vi "VASP Helper.vi"() -> ()   [LabVIEW 2010]
uses:
  <vilib>/Utility/miscctls.llb/LV3DPointTypeDef.ctl
  <vilib>/addons/database/_DB Variant To Data/Database Variant To Data.xnode
  <vilib>/Analysis/6fits.llb/Curve Fitting Criteria.ctl
  <vilib>/Analysis/_algsub.llb/Real Vector Norm.vi
  <vilib>/Utility/file.llb/Read From Spreadsheet File (string).vi
  <vilib>/addons/database/Connection.llb/DB Tools Open Connec (Path).vi
  <vilib>/gmath/NumericalOptimization/Nonlinear Curve Fit LM formula string.vi
  <vilib>/Utility/file.llb/Write To Spreadsheet File (string).vi
  <vilib>/Analysis/NI_AALPro.lvlib
  <vilib>/addons/database/NI_Database_API.lvlib
  <vilib>/picture/3D Picture Control/NI_3D Picture Control.lvlib
  <vilib>/gmath/NI_Gmath.lvlib
panel:
  in  "Bulk Stds":T1(array[cluster])=[{"Bulk Name"="Relax2", "Structure ID"="i8VcOVQciOra", "Final Energy (eV)"=-19.916802, "Atom Counts"=[{"Atomic Species"="Cd", "Total Count"=4}, {"Atomic Species"="Te", "Total Count"=4}]}, {"Bulk Name"="Gamma8_64atom", "Structure ID"="KHRErLzu78i1", "Final Energy (eV)"=-159.32149, "Atom Counts"=[{"Atomic Species"="Cd", "Total Count"=32}, {"Atomic Species"="Te", "Total Count"=32}]}, {"Bulk Name"="Gamma8_216atom", "Structure ID"="LhCMwqUcPen4", "Final Energy (eV)"=-537.73861, "Atom Counts"=[{"Atomic Species"="Cd", "Total Count"=108}, {"Atomic Species"="Te", "Total Count"=108}]}, {"Bulk Name"="Gamma8_111Bulk", "Structure ID"="Ku1Zi1Vogv1V", "Final Energy (eV)"=-29.865487, "Atom Counts"=[{"Atomic Species"="Cd", "Total Count"=6}, {"Atomic Species"="Te", "Total Count"=6}]}, {"Bulk Name"="A3B3_Supercell_C+0.147672", "Structure ID"="F1CSD7Lr82d2", "Final Energy (eV)"=-358.27975, "Atom Counts"=[{"Atomic Species"="Cd", "Total Count"=72}, {"Atomic Species"="Te", "Total Count"=72}]}, {"Bulk Name"="A4B1_Supercell_C+0.130973", "Structure ID"="gulg5TYIiUnY", "Final Energy (eV)"=-298.52824, "Atom Counts"=[{"Atomic Species"="Cd", "Total Count"=60}, {"Atomic Species"="Te", "Total Count"=60}]}]
  out "IDs":T2
  out "Temp Interfacial Area":dbl
  out "Temp # of atoms":i32
  out "Temp Values":string[](array[string])
  out "Temp Headers":string[](array[string])
  out "Using DB":bool
  out "Selected DOS":T3
  out "DOS Array":T4(array[cluster])
  out "Selected Structure":T5
  out "PickPoint":T6
  out "DOS Plot Names":string[](array[string])
  out "Saved DOS Plots":cluster{dbl[], dbl[]}[](array[cluster])
  in  "Plot Formation Energy":bool
  in  "Plot Band Edge Diagram":bool=TRUE
  in  "Plot Bivariate":bool=TRUE
  in  "Save Summary":bool
  in  "Plot Structures":bool
  in  "Primary Path":path
  in  "Clean Cache":bool
  in  "Loaded DFT Paths":path[](array[path])
  out "OSZICAR Raw Array":T7(array[cluster])
  out "All DFT Data Summary":T8
  in  "Plot Relaxation":bool
  in  "Plot DOS":bool
  in  "Plot Variability":bool
  in  "Load from DB":bool
  in  "Load from Directory":bool
  in  "Details":i32[](listbox)
  in  "Selection List":i32[](listbox)
  in  "Tab Control":T9(tab)
  out "Overview DOS PLot":cluster{dbl[], dbl[]}[](graph)
  out "Overview - Relaxation":cluster{"Formation Energy (eV)":dbl[]}[](graph)
  out "Overview - Parameter Analysis Graph":cluster{"Voltage":dbl[], dbl[]}[](graph)=[{"Voltage"=[], []}, {"Voltage"=[1.0], [nan]}]
  out "Relaxation":cluster{"Formation Energy (eV)":dbl[]}[](graph)
  in  "Relaxation Y-Axis":string(combo)="Energy"
  in  "Send to DOS":bool
  in  "Load in VESTA":bool
  in  "Auto Setup Camera":bool
  out "Atomic Structure":refnum<vi>(3d-picture)
  in  "Animate Relaxation":bool
  in  "Atom Size":dbl=0.75
  in  "# Frames":i32(slide)=5 scale=0.0..100.0
  in  "Atom List":i32[](listbox)
  in  "Scale":dbl(slide)=0.07482993197278912 scale=0.0..0.5
  in  "CONTCAR?":bool
  in  "Look at Atoms":bool
  in  "Plot Name":string
  in  "Erase":bool
  in  "DOS Sum and Plot":bool
  in  "DOS Options":i32[](listbox)
  in  "Always Show Bulk":bool
  out "DOS PLot":cluster{dbl[], dbl[]}[](graph)
  in  "S Orbitals":bool
  in  "P Orbital":bool
  in  "D Orbitals":bool
  out "Band Edge Diagram":cluster{"Array":dbl[], dbl[]}[](graph)
  in  "Low Density Cutoff":dbl
  in  "Style":enum16{"Linear Step", "Linear Pts", "Log Pts"}(ring)
  in  "Step or #pts":dbl
  in  "Grouping Columns":u16[](array[ring])=[2] items=["Full_Directory", "Parent_Folder", "Folder", "# Atoms", "Cell Volume (A^3)", "|A| (Å)", "|B| (Å)", "|C| (Å)", "alpha (deg)", "beta (deg)", "gamma (deg)", "Final_Energy_(eV)", "Final Energy/atom (eV/atom)", "Total Formation Energy (eV)", "E0 at Sigma=0 (eV)", "dE (eV)", "Interfacial Energy (J/m²)", "Calc Time (hrs)", "Grain 1 Orientation", "Grain 2 Orientation", "Twist Angle (Degree)", "Tilt Angle (Degree)", "Translation (x,y,z)", "Overlap Length (A)", "Grain 1 Start (A)", "Defect Name", "Location"]
  in  "Parameter Analysis Y-Axis":u16(ring)=23 caption="| Current Density | (A/cm2)" items=["Full_Directory", "Parent_Folder", "Folder", "# Atoms", "Cell Volume (A^3)", "|A| (Å)", "|B| (Å)", "|C| (Å)", "alpha (deg)", "beta (deg)", "gamma (deg)", "Final_Energy_(eV)", "Final Energy/atom (eV/atom)", "Total Formation Energy (eV)", "E0 at Sigma=0 (eV)", "dE (eV)", "Interfacial Energy (J/m²)", "Calc Time (hrs)", "Grain 1 Orientation", "Grain 2 Orientation", "Twist Angle (Degree)", "Tilt Angle (Degree)", "Translation (x,y,z)", "Overlap Length (A)", "Grain 1 Start (A)", "Defect Name", "Location"]
  out "Parameter Analysis Graph":cluster{"Voltage":dbl[], dbl[]}[](graph)=[{"Voltage"=[], []}, {"Voltage"=[1.0], [nan]}]
  in  "model description":T10
  out "best fit parameters":dbl[](array[numeric])
  in  "initial parameters":dbl[](array[numeric])
  out "R²":dbl
  out "X_min":dbl
  in  "Bivariate X-Axis":string(combo)="Energy"
  in  "Bivariate Y-Axis":string(combo)="Energy"
  out "Bivariate Plot":cluster{dbl[], dbl[]}[](graph)
  out "Ymin":dbl
  out "Polynomial Coefficients":dbl[](array[numeric])
  in  "Standard Bulk Calculations":i32[](listbox)
  in  "Add to point defect DB":bool
  out "Te Rich Limit":cluster{"appended array":dbl[], dbl[]}[](graph)
  out "Reference Energy (eV)":dbl format="%#_6f"
  out "Cd Rich Limit":cluster{"appended array":dbl[], dbl[]}[](graph)
  in  "Add to README files":bool
  in  "Loaded Files":i32[](listbox)
  in  "Size Factor":i32=1
  out "GB Bivariate Plot":cluster{dbl[], dbl[]}(graph)
  in  "Interface Free Reference Energy":i32[](listbox)
  in  "GB Size Factor":dbl=1.0
  out "GB Reference Energy (eV)":dbl
  in  "Add to GB DB":bool
  in  "Color Array Type":T11(ring)=enum."Contrasting Colors"
  in  "Load Energies":bool=TRUE
  in  "Load DOS":bool=TRUE
  in  "Only total DOS":bool=TRUE
  out "Structures":T12(array[cluster])
  out "All Available DFT Paths":path[](array[path])
  in  "Vesta .exe Location":path=path "C:/Program Files (x86)/VESTA/VESTA.exe"
  out "Selectd Defect Data":T13(array[cluster])
  out "Base Object":refnum<vi>
  in  "Vasp DB UDL":path=path "D:/Ab-initio/VASP Calcs/VASP DB.udl"
  in  "Options":cluster{"Border?":bool, "Bonds?":bool}={"Border?"=TRUE, "Bonds?"=FALSE}
  # "After"
  # "Before"
  # "You need non self-cons"
  # "Most Specific"
  # "Least Specific"
  # "Interface at b*c"
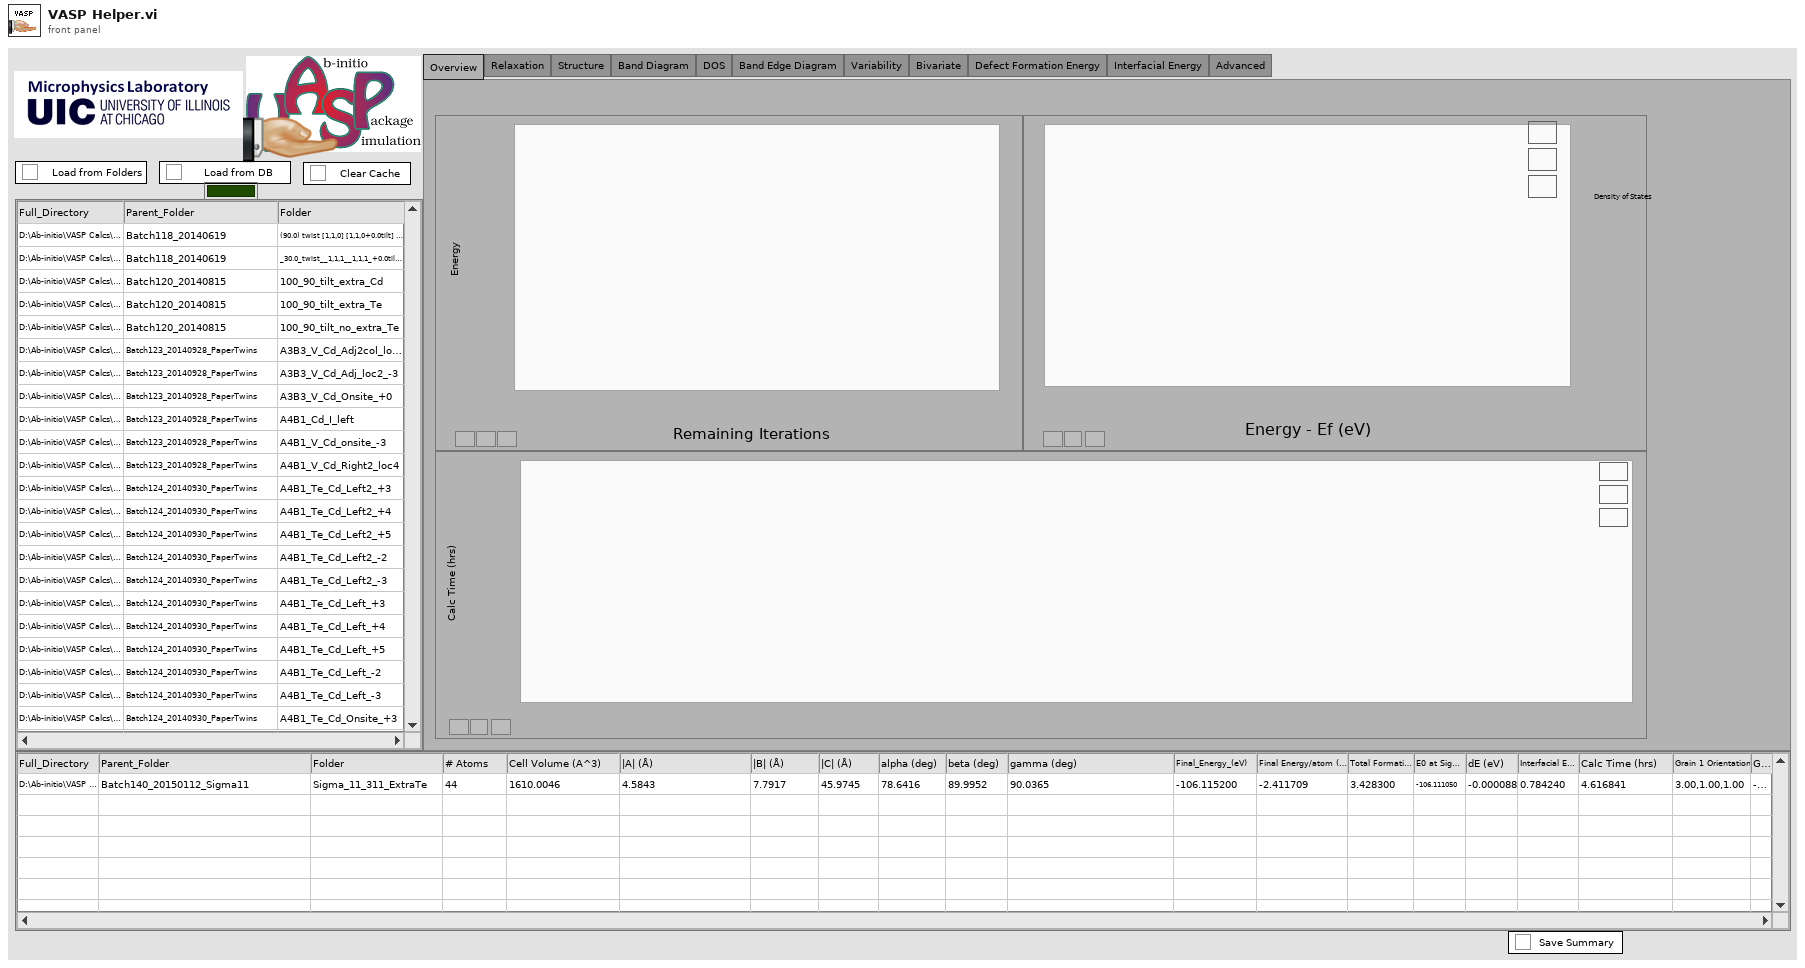
[diagram p1: front panel]
types:
  T1 = cluster{"Bulk Name":string, "Structure ID":string, "Final Energy (eV)":dbl, "Atom Counts":cluster{"Atomic Species":string, "Total Count":i32}[]}[]
  T2 = cluster{"CONTCAR ID":string, "OSZICAR ID":string, "DOSCAR ID":string}
  T3 = cluster{"DOS Summary":cluster{"Fermi Level (eV)":dbl, "# Filled States":dbl, "Density of Valence Band":dbl, "Density of Condution Band":dbl}, "Total DOS":cluster{"Energy (eV)":dbl[], "Total DOS":dbl[], "Integrated DOS":dbl[]}, "Atomic-decomposed DOS":cluster{"Fermi Level (eV)":dbl, "# of Filled States":dbl, "DOS":dbl[][]}[]}
  T4 = cluster{"DOS Summary":cluster{"Fermi Level (eV)":dbl, "# Filled States":dbl, "Density of Valence Band":dbl, "Density of Condution Band":dbl}, "Total DOS":cluster{"Energy (eV)":dbl[], "Total DOS":dbl[], "Integrated DOS":dbl[]}, "Atomic-decomposed DOS":cluster{"Fermi Level (eV)":dbl, "# of Filled States":dbl, "DOS":dbl[][]}[]}[]
  T5 = cluster{"Structure Name":string, "Lattice vector a":dbl[], "Lattice vector b":dbl[], "Lattice vector c":dbl[], "Atoms Array":cluster{"Atom Name":string, "Positions (Direct)":dbl[][], "Positions (Cartesian)":dbl[][]}[], "# of atoms":i32}
  T6 = typedef "LV3DPointTypeDef.ctl" = cluster{"X":sgl, "Y":sgl, "Z":sgl}
  T7 = cluster{"OSZICAR data":cluster{"Total Free Energy (eV)":dbl, "E0 at Sigma=0 (eV)":dbl, "dE (eV)":dbl, "Electronic Relaxation":dbl[][]}[], "Ionic Relaxation Energies Array (eV)":dbl[], "Bulk Formation Energies Array (eV)":dbl[]}[]
  T8 = cluster{"Headers":string[], "Relaxation Data":string[][]}
  T9 = enum32{"Overview", "Relaxation", "Structure", "Band Diagram", "DOS", "Band Edge Diagram", "Variability", "Bivariate", "Defect Formation Energy", "Interfacial Energy", "Advanced"}
  T10 = cluster{"model":string, "Parameters":string[], "x":string}
  T11 = enum16{"Visible Spectrum", "Greyscale", "Contrasting Colors"}
  T12 = cluster{"Structure Name":string, "Lattice vector a":dbl[], "Lattice vector b":dbl[], "Lattice vector c":dbl[], "Atoms Array":cluster{"Atom Name":string, "Positions (Direct)":dbl[][], "Positions (Cartesian)":dbl[][]}[], "# of atoms":i32}[]
  T13 = cluster{"Final Total Defect Energy (eV)":dbl, "Reference Pure Structure Energy":dbl, "N (Cd,Ideal - Cd,Defect)":i32, "N (Te,ideal - Te,defect)":i32, "# Extra Electrons":i32}[]
  T14 = cluster{"DOS Summary":cluster{"Fermi Level (eV)":dbl, "# States":dbl, "Density of Valence Band":dbl, "Density of Condution Band":dbl}, "Total DOS":cluster{"Energy (eV)":dbl[], "Total DOS":dbl[], "Integrated DOS":dbl[]}, "Atomic-decomposed DOS":cluster{"Fermi Level (eV)":dbl, "# of Filled States":dbl, "DOS":dbl[][]}[]}[]
  T15 = enum32{"Overview", "Relaxation", "Structure", "Band Diagram", "DOS", "Band Edge Diagram", "Variability", "Bivariate", "Defect Formation Energy", "Advanced"}
  T16 = cluster{"OSZICAR data":cluster{"Total Free Energy (eV)":dbl, "E0 at Sigma=0 (eV)":dbl, "dE (eV)":dbl, "Electronic Relaxation":dbl[][]}[], "Ionic Relaxation Energies Array (eV)":dbl[], "Bulk Formation Energies Array (eV)":dbl[]}
  T17 = cluster{"Final Energy (eV)":dbl, "Final Energy/atom (eV/atom)":dbl, "Total Formation Energy (eV)":dbl}
  T18 = cluster{"Fermi Level (eV)":dbl, "# of Filled States":dbl, "DOS":dbl[][]}[]
  T19 = cluster{"Energy (eV)":dbl[], "Total DOS":dbl[], "Integrated DOS":dbl[]}
  T20 = cluster{"Fermi Level (eV)":dbl, "# States":dbl, "Density of Valence Band":dbl, "Density of Condution Band":dbl}
  T21 = cluster{"DOS Summary":cluster{"Fermi Level (eV)":dbl, "# States":dbl, "Density of Valence Band":dbl, "Density of Condution Band":dbl}, "Total DOS":cluster{"Energy (eV)":dbl[], "Total DOS":dbl[], "Integrated DOS":dbl[]}, "Atomic-decomposed DOS":cluster{"Fermi Level (eV)":dbl, "# of Filled States":dbl, "DOS":dbl[][]}[]}
  T22 = typedef "NI_Database_API.lvlib/Conn ObjectReference.ctl" = refnum<k1>
  T23 = cluster{"[0]":string, "[1]":string, "[2]":string}
  T24 = cluster{"Bulk Formation Energies Array (eV)":dbl[]}
  T25 = cluster{"Atom Name":string, "Positions (Direct)":dbl[][], "Positions (Cartesian)":dbl[][]}[]
  T26 = cluster{"Fermi Level (eV)":dbl, "# of Filled States":dbl, "DOS":dbl[][]}
  T27 = typedef "NI_AALPro.lvlib/Curve Fitting Criteria.ctl" = u16
  T28 = cluster{"Lattice vector b[0]":dbl, "Lattice vector b[1]":dbl, "Lattice vector b[2]":dbl}
  T29 = typedef "LVPoint32TypeDef.ctl" = cluster{"Horizontal":i32, "Vertical":i32}
  T30 = cluster{"Shift":bool, "Ctrl":bool, "Alt":bool, "Cmd":bool, "Opt":bool}
  T31 = typedef "LVPositionTypeDef.ctl" = cluster{"Left":i32, "Top":i32}
  T32 = cluster{"Bulk Name":string, "Structure ID":string, "Final Energy (eV)":dbl, "Atom Counts":cluster{"Atomic Species":string, "Total Count":i32}[]}
  T33 = cluster{"Atomic Species":string, "Total Count":i32}[]
  T34 = cluster{"String":string, string, dbl, "Atom Counts":cluster{"Atomic Species":string, "Total Count":i32}[]}
  T35 = cluster{"Atomic Species":string, "Total Count":i32}
  T36 = cluster{"String":string, "Site Density":dbl, dbl, i32, i32}
  T37 = cluster{cluster{"String":string, "Site Density":dbl, dbl, i32, i32}, cluster{string, string, "Net Charge":i32, dbl}[]}
  T38 = cluster{"String":string, "Structure ID":string, "String":string, "String":string, i32, "Structure ID":string, "name":string, "Reference Pure Structure Energy":dbl, "N (Cd,Ideal - Cd,Defect)":i32, "N (Te,ideal - Te,defect)":i32, string}
  T39 = cluster{"DFT ID":string, "Structure ID":string, "Defect_Name":string, "Location":string, "Net Charge":i32, "Defect Free Structure ID":string, "Defect Free Structure Name":string, "Reference Pure Structure Energy":dbl, "N Mising Cd":i32, "N Missing Te":i32, "Comments":string}[]
  T40 = cluster{"MD5 message-digest":string, "Structure ID":string, "String":string, "Structure ID":string, "name":string, "GB Reference Energy (eV)":dbl, "t":dbl, dbl, dbl, "String":string, string}
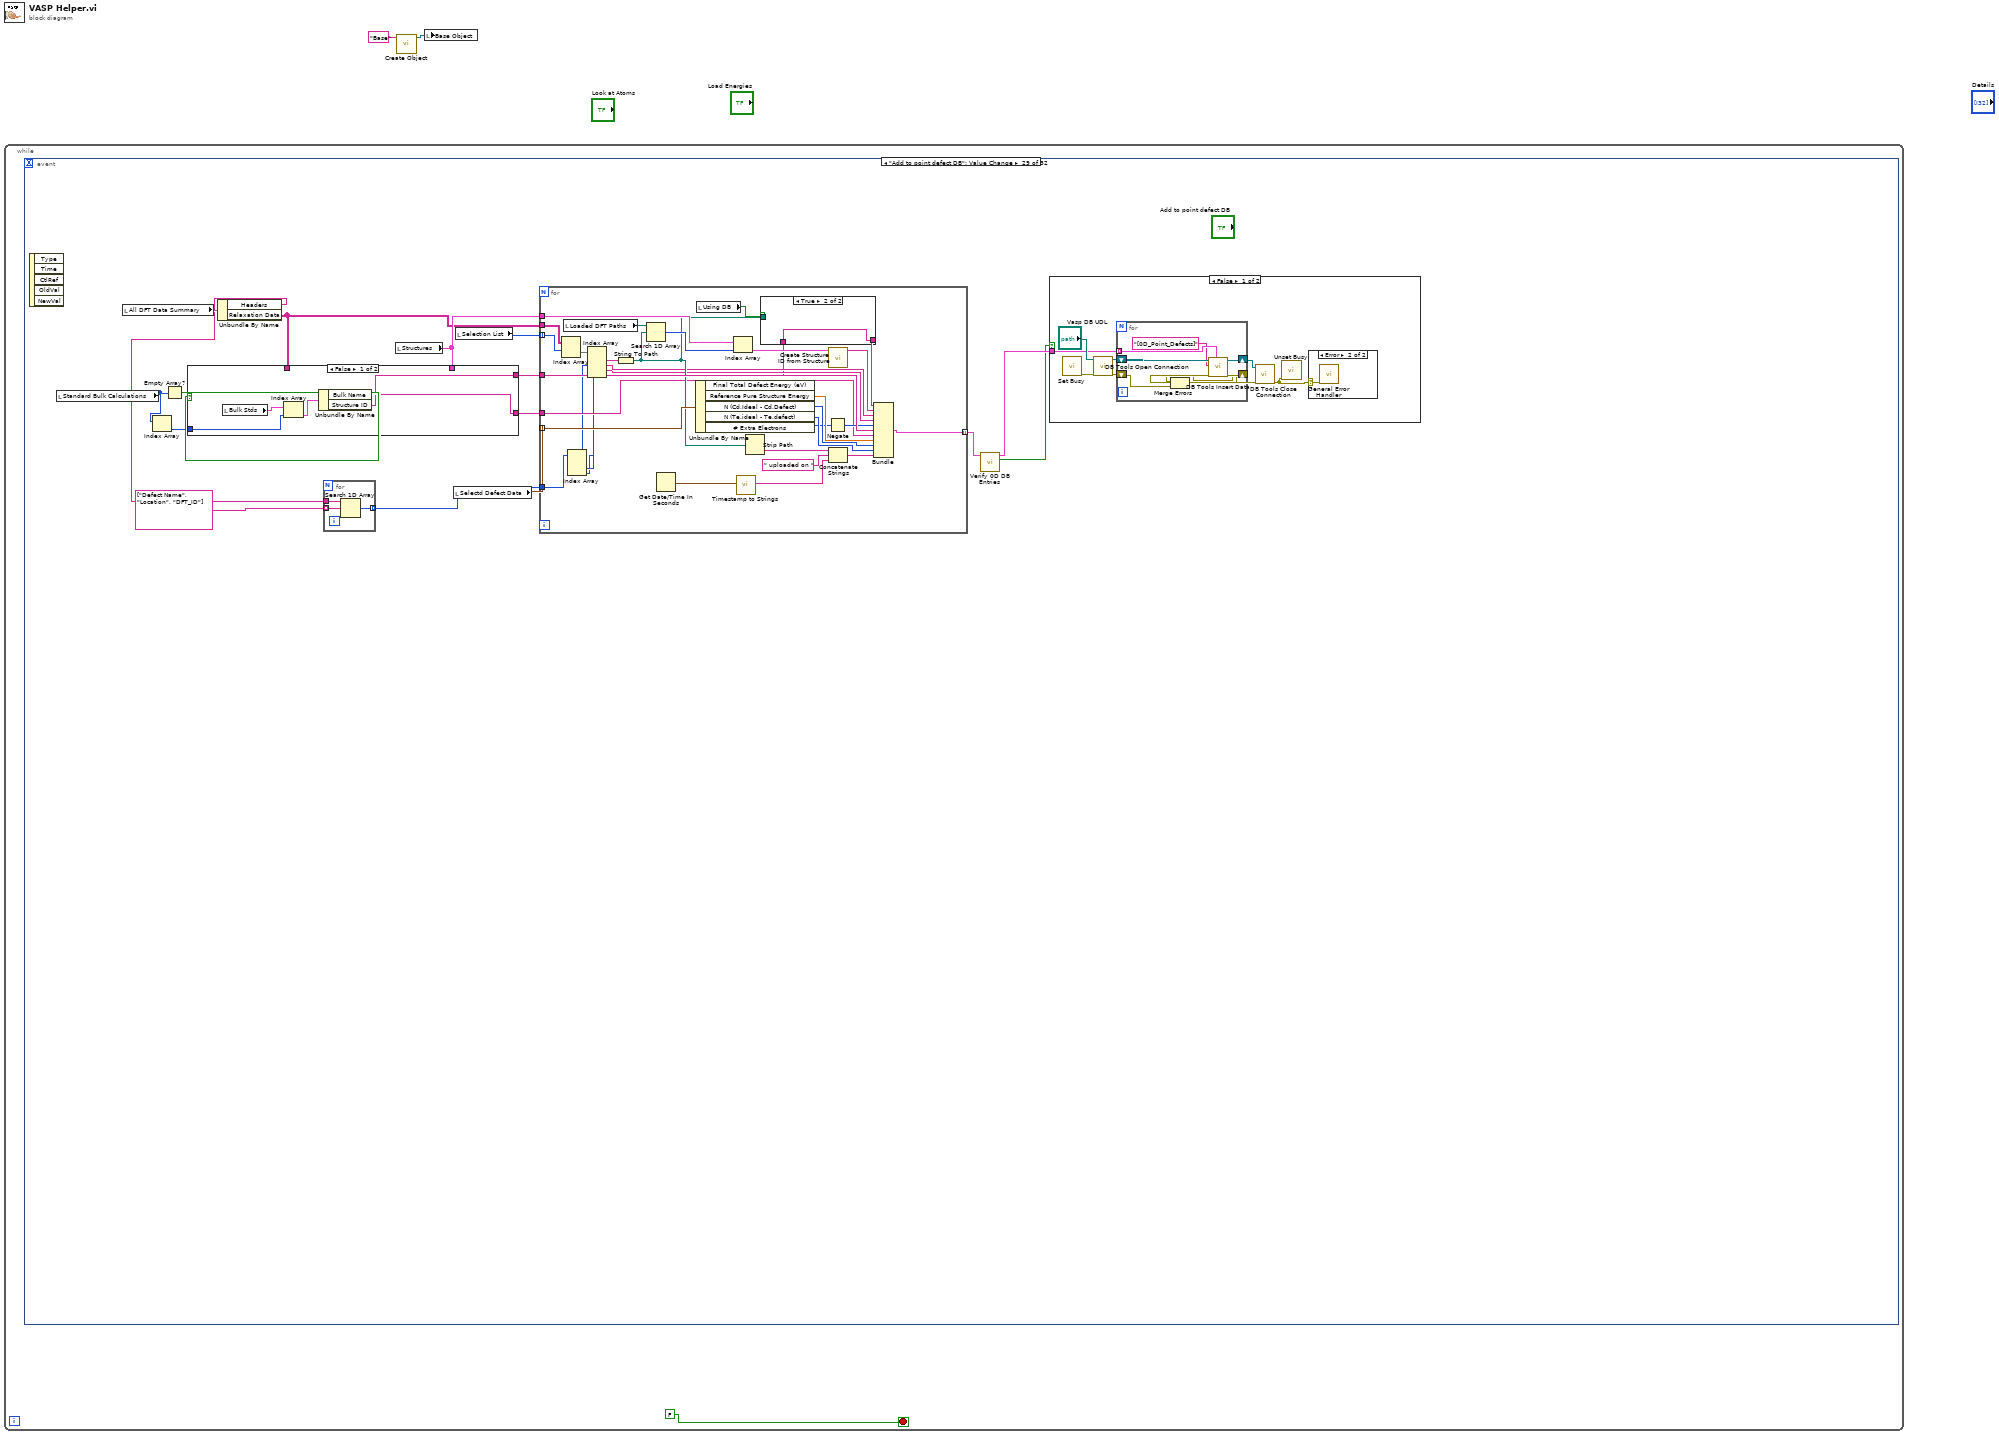
[diagram p0: block diagram]
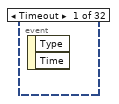
[diagram p2: hidden frame]
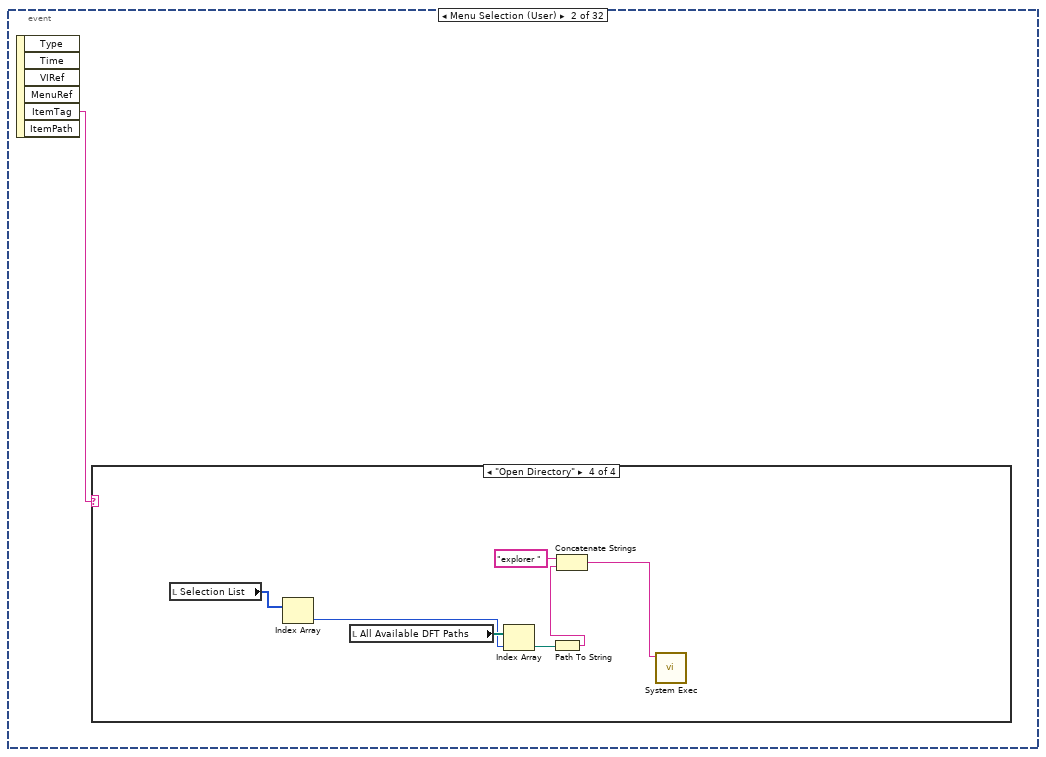
[diagram p3: hidden frame]
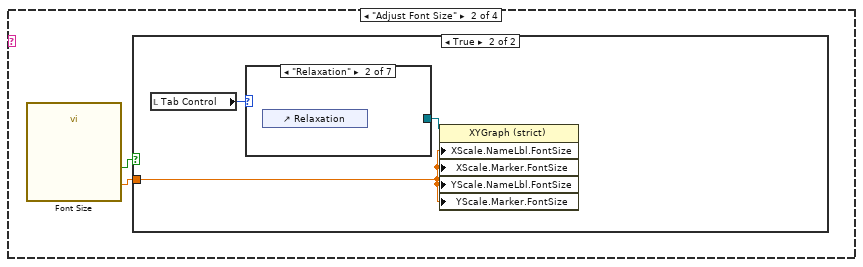
[diagram p5: hidden frame]
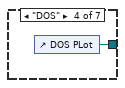
[diagram p9: hidden frame]
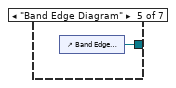
[diagram p10: hidden frame]
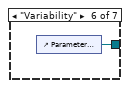
[diagram p11: hidden frame]
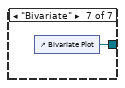
[diagram p12: hidden frame]
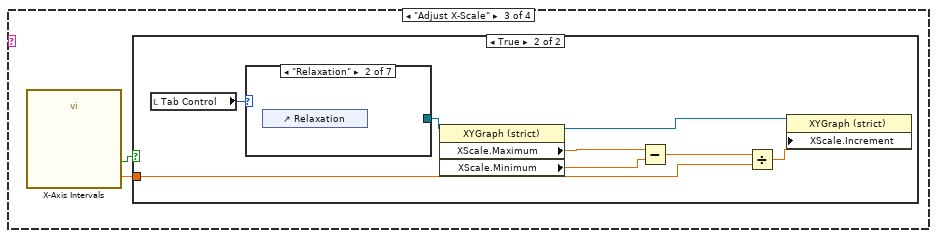
[diagram p13: hidden frame]
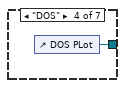
[diagram p17: hidden frame]
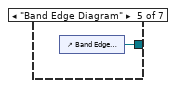
[diagram p18: hidden frame]
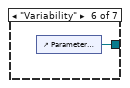
[diagram p19: hidden frame]
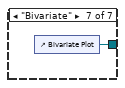
[diagram p20: hidden frame]
diagram:
  n1 = while {
    stop <- FALSE stop-if-true
    n2 = event shown="[28] \"Add to point defect DB\": Value Change" {
      selector: _ -> [_ _ _ _ _ _ _ _ _ _ _ _ _ _ _ _ _ _ _ _ _ _ _ _ _ _ _ _ _ _ _ _]
      dyn-events: _ -> [_ _ _ _ _ _ _ _ _ _ _ _ _ _ _ _ _ _ _ _ _ _ _ _ _ _ _ _ _ _ _ _]
      timeout: _ -> [_ _ _ _ _ _ _ _ _ _ _ _ _ _ _ _ _ _ _ _ _ _ _ _ _ _ _ _ _ _ _ _]
      event Timeout {
        n3 = event-data() -> ()  [unwired: 1 in, 2 out]
      }
      event Menu Selection (User) {
        n4 = event-data() -> ("ItemTag"=w4:string)  [unwired: 1 in, 5 out]
        n5 = case shown="\"Open Directory\"" w4 {
          frame Default {
          }
          frame "Adjust Font Size" {
            n6 = call "Font Size"() -> ("Font Size"=w5:dbl, "Apply"=w6:bool)  [unwired: 17 in, 1 out]
            n7 = case shown="True" w6 {
              tunnel: w5 -> [_ w9]
              frame False {
              }
              frame True {
                n8 = local read "Tab Control"() -> (w8:T9)
                n9 = case shown="\"Relaxation\"" w8 {
                  tunnel: [_ _ _ w10 w11 w12 w13] -> w7
                  frame "Overview", Default {
                  }
                  frame "Relaxation" {
                    n10 = control-ref of="Relaxation"() -> ()  [unwired: 1 out]
                  }
                  frame "Structure" {
                  }
                  frame "DOS" {
                    n11 = control-ref of="DOS PLot"() -> (w10:refnum<vi>)
                  }
                  frame "Band Edge Diagram" {
                    n12 = control-ref of="Band Edge Diagram"() -> (w11:refnum<vi>)
                  }
                  frame "Variability" {
                    n13 = control-ref of="Parameter Analysis Graph"() -> (w12:refnum<vi>)
                  }
                  frame "Bivariate" {
                    n14 = control-ref of="Bivariate Plot"() -> (w13:refnum<vi>)
                  }
                }
                n15 = property on="Property Node" class="XYGraph (strict)"(reference=w7, "XScale.NameLbl.FontSize"=w9, "XScale.Marker.FontSize"=w9, "YScale.NameLbl.FontSize"=w9, "YScale.Marker.FontSize"=w9) -> ()  [unwired: 1 in, 2 out]
              }
            }
          }
          frame "Adjust X-Scale" {
            n16 = call "X-Axis Intervals"() -> ("# Intervals"=w14:dbl, "Apply"=w15:bool)  [unwired: 17 in, 1 out]
            n17 = case shown="True" w15 {
              tunnel: w14 -> [_ w19]
              frame False {
              }
              frame True {
                n18 = local read "Tab Control"() -> (w23:T9)
                n19 = case shown="\"Relaxation\"" w23 {
                  tunnel: [_ _ _ w24 w25 w26 w27] -> w17
                  frame "Overview", Default {
                  }
                  frame "Relaxation" {
                    n20 = control-ref of="Relaxation"() -> ()  [unwired: 1 out]
                  }
                  frame "Structure" {
                  }
                  frame "DOS" {
                    n21 = control-ref of="DOS PLot"() -> (w24:refnum<vi>)
                  }
                  frame "Band Edge Diagram" {
                    n22 = control-ref of="Band Edge Diagram"() -> (w25:refnum<vi>)
                  }
                  frame "Variability" {
                    n23 = control-ref of="Parameter Analysis Graph"() -> (w26:refnum<vi>)
                  }
                  frame "Bivariate" {
                    n24 = control-ref of="Bivariate Plot"() -> (w27:refnum<vi>)
                  }
                }
                n25 = property on="Property Node" class="XYGraph (strict)"(reference=w17) -> (reference out=w16:refnum<vi>, "XScale.Maximum"=w22:dbl, "XScale.Minimum"=w21:dbl)  [unwired: 1 in, 1 out]
                n26 = Subtract(x=w22, y=w21) -> (x-y=w20:dbl)
                n27 = Divide(x=w20, y=w19) -> (x/y=w18:dbl)
                n28 = property on="Property Node" class="XYGraph (strict)"(reference=w16, "XScale.Increment"=w18) -> ()  [unwired: 1 in, 2 out]
              }
            }
          }
          frame "Open Directory" {
            n29 = local read "Selection List"() -> (w33:i32[])
            n30 = Index Array(array=w33) -> (element=w32:i32)  [unwired: 1 in]
            n31 = local read "All Available DFT Paths"() -> (w34:path[])
            n32 = Index Array(array=w34, index=w32) -> (element=w28:path)
            n33 = Path To String(path=w28) -> (string=w31:string)
            n34 = Concatenate Strings("explorer " ("string"), w31) -> (w29:string)
            n35 = call <vilib>:"System Exec.vi"("command line"=w29) -> ()  [unwired: 7 in, 4 out]
          }
        }
      }
      event "Primary Path", "Load from Directory": Value Change {
        w35 = string[] ["Full_Directory", "Parent_Folder", "Folder"]
        n36 = event-data() -> ()  [unwired: 1 in, 5 out]
        n37 = call "File Dialog2"("start path"=path "D:/Ab-initio/VASP Calcs" ("Folder Path"), "prompt"="Please choose the primary path where all VASP calculation folders are stored.\nThis will be done recursively") -> ("selected path"=w40:path)  [unwired: 10 in, 3 out]
        n38 = flat-sequence {
          frame #0 {
            n39 = local write "Loaded DFT Paths"(path[] [] ("Loaded DFT Paths")) -> ()
            n40 = local write "OSZICAR Raw Array"(T7 [] ("OSZICAR Raw Array")) -> ()
            n41 = local write "DOS Array"(T14 [] ("DOS Array")) -> ()
            n42 = local write "Structures"(T12 [] ("Structures")) -> ()
            n43 = Request Deallocation(TRUE ("flag")) -> ()
          }
        }
        n44 = local write "Primary Path"(w40) -> ()
        n45 = call <vilib>:"Recursive File List.vi"("Folder Path"=w40) -> ("All Folders"=w45:path[])  [unwired: 6 in, 4 out]
        n46 = for {
          tunnel: w45 -> [w55] mode=indexing
          shift-right: [w54] -> w41
          shift-left: path[] [] -> [w53]
          shift-right: [w52] -> w36
          shift-left: string[][] [] -> [w51]
          n47 = Build Path(base path=w55, name or relative path="POSCAR") -> (appended path=w57:path)
          n48 = call <vilib>:"Check if File or Folder Exists.vi"("path"=w57) -> ("file or folder exists?"=w56:bool)  [unwired: 8 in, 2 out]
          n49 = case shown="False" w56 {
            tunnel: w55 -> [_ w67]
            tunnel: [w60 w70] -> w54
            tunnel: w53 -> [w60 w69]
            tunnel: [w59 w62] -> w52
            tunnel: w51 -> [w59 w61]
            frame False {
            }
            frame True {
              n50 = Build Array (concatenate)(w69, w67) -> (w70:path[])
              n51 = Strip Path(path=w67) -> (stripped path=w66:path, name=w65:string)
              n52 = Path To String(path=w67) -> (string=w68:string)
              n53 = Strip Path(path=w66) -> (name=w64:string)  [unwired: 1 out]
              n54 = Build Array(w68, w64, w65) -> (w63:string[])
              n55 = Build Array (concatenate)(w61, w63) -> (w62:string[][])
            }
          }
        }
        "All Available DFT Paths" <- w41
        n56 = local write "Using DB"(FALSE ("Using DB")) -> ()
        n57 = property on="Selection List" class="MCListbox (strict)"("ColHdrString"=w35, "ItemNames"=w36) -> ()  [unwired: 2 in, 2 out]
        n58 = Bundle(w35, w36) -> (w42:cluster{string[], string[][]})  [unwired: 1 in]
        n59 = local write "All DFT Data Summary"(w42) -> ()
        n60 = property on="Loaded Files" class="MCListbox (strict)"("ItemNames"=w36) -> ()  [unwired: 2 in, 2 out]
        n61 = property on="Interface Free Reference Energy" class="MCListbox (strict)"("ColHdrString"=w35, "ItemNames"=w36) -> ()  [unwired: 2 in, 2 out]
      }
      event "Load from DB": Value Change {
        n62 = event-data() -> ()  [unwired: 1 in, 5 out]
        n63 = flat-sequence {
          frame #0 {
            n64 = local write "Loaded DFT Paths"(path[] [] ("Loaded DFT Paths")) -> ()
            n65 = local write "OSZICAR Raw Array"(T7 [] ("OSZICAR Raw Array")) -> ()
            n66 = local write "DOS Array"(T14 [] ("DOS Array")) -> ()
            n67 = local write "Structures"(T12 [] ("Structures")) -> ()
            n68 = Request Deallocation(TRUE ("flag")) -> ()
          }
        }
        n69 = call "Import from VASP DB.vi"() -> ("error out"=w74:errorcluster, "All DFT Data Summary"=w78:T8)  [unwired: 10 in]
        n70 = local write "All DFT Data Summary"(w78) -> ()
        n71 = Unbundle(w78) -> ("Headers"=w71:string[], "Relaxation Data"=w72:string[][])
        n72 = property on="Selection List" class="MCListbox (strict)"("ColHdrString"=w71, "ItemNames"=w72) -> ()  [unwired: 2 in, 2 out]
        n73 = property on="Loaded Files" class="MCListbox (strict)"("ItemNames"=w72) -> ()  [unwired: 2 in, 2 out]
        n74 = property on="Details" class="MCListbox (strict)"("ColHdrString"=w71) -> ()  [unwired: 2 in, 2 out]
        n75 = Index Array(array=w72, index (col)=0 ("disabled index (col)")) -> (element=w76:string[])  [unwired: 1 in]
        n76 = for {
          tunnel: w76 -> [w85] mode=indexing
          tunnel: [w84] -> w75 mode=indexing
          tunnel: w74 -> [_]
          n77 = String To Path(string=w85) -> (path=w84:path)
        }
        n78 = property on="Interface Free Reference Energy" class="MCListbox (strict)"("ColHdrString"=w71, "ItemNames"=w72) -> ()  [unwired: 2 in, 2 out]
        n79 = local write "All Available DFT Paths"(w75) -> ()
        "Using DB" <- TRUE ("Using DB")
      }
      event "Selection List": Value Change {
        n80 = event-data() -> ()  [unwired: 1 in, 5 out]
        n81 = for {
          tunnel: [w98] -> w86 mode=indexing
          tunnel: "Selection List" -> [w95] mode=indexing
          tunnel: [w92] -> w87
          n82 = local read "All Available DFT Paths"() -> (w93:path[])
          n83 = Index Array(array=w93, index=w95) -> (element=w96:path)
          n84 = Search 1D Array(1D array="Loaded DFT Paths", element=w96) -> (index of element=w97:i32)  [unwired: 1 in]
          n85 = case shown="-1" w97 {
            tunnel: [w100 w106] -> w98
            tunnel: w96 -> [_ w107]
            tunnel: w95 -> [w101 w108]
            tunnel: [w99 w105] -> w92
            frame Default {
              n86 = local read "All DFT Data Summary"() -> (w103:T8)
              n87 = Unbundle By Name(w103) -> ("Headers"=w99:string[], "Relaxation Data"=w102:string[][])
              n88 = Index Array(array=w102, index (row)=w101) -> (element=w100:string[])  [unwired: 1 in]
            }
            frame -1 {
              n89 = local read "Using DB"() -> (w104:bool)
              n90 = case shown="True" w104 {
                tunnel: w108 -> [w112 w222]
                tunnel: w107 -> [w111 w225]
                tunnel: [w110 w223] -> w106
                tunnel: [w109 w224] -> w105
                frame False {
                  n91 = stacked-sequence {
                    tunnel: w112 -> [_ _ _ _ _ _ _ w213]
                    tunnel: w111 -> [w115 w119 w141 w166 w176 w179 w199 _]
                    tunnel: [_ _ _ _ _ _ _ w209] -> w110
                    tunnel: [_ _ _ _ _ _ _ w210] -> w109
                    tunnel: [_ _ _ _ w168 _ _ _] -> _
                    frame #0 {
                      w113 = string[] [] ("Temp Headers")
                      # "Add new path to list"
                      n92 = local read "Loaded DFT Paths"() -> (w116:path[])
                      n93 = local write "Temp Headers"(w113) -> ()
                      n94 = local write "Temp Values"(w113) -> ()
                      n95 = Build Array (concatenate)(w116, w115) -> (w114:path[])
                      n96 = local write "Loaded DFT Paths"(w114) -> ()
                    }
                    frame #1 {
                      n97 = Strip Path(path=w119) -> (stripped path=w127:path, name=w124:string)
                      n98 = Path To String(path=w119) -> (string=w126:string)
                      n99 = Strip Path(path=w127) -> (name=w125:string)  [unwired: 1 out]
                      n100 = Build Array(w126, w125, w124) -> (w121:string[])
                      n101 = local read "Temp Headers"() -> (w123:string[])
                      n102 = local read "Temp Values"() -> (w122:string[])
                      n103 = Build Array (concatenate)(w123, string[] ["Full_Directory", "Parent_Folder", "Folder"]) -> (→"Temp Headers":string[])
                      n104 = Build Array (concatenate)(w122, w121) -> (→"Temp Values":string[])
                    }
                    frame #2 {
                      n105 = Build Path(base path=w141, name or relative path="CONTCAR") -> (appended path=w144:path)
                      n106 = call "Parse POSCAR.vi"("POSCAR File"=w144) -> ("Summary Values"=w136:string[], "Summary Headers"=w137:string[], "Structure"=w131:T5)  [unwired: 7 in, 1 out]
                      n107 = Unbundle By Name(w131) -> ("Lattice vector a"=w134:dbl[], "Lattice vector b"=w133:dbl[], "# of atoms"=→"Temp # of atoms":i32)
                      n108 = local read "Temp Headers"() -> (w138:string[])
                      n109 = local read "Temp Values"() -> (w140:string[])
                      n110 = local read "Structures"() -> (w142:T12)
                      n111 = call <vilib>:"Cross Product.vi"("B Vector"=w133, "A Vector"=w134) -> ("Cross Product"=w132:dbl[])  [unwired: 8 in, 1 out]
                      n112 = call-poly <vilib>:"Vector Norm.vi"("Input Vector"=w132) -> ("norm"=→"Temp Interfacial Area":dbl)  [unwired: 9 in, 1 out]
                      n113 = Build Array (concatenate)(w142, w131) -> (→"Structures":T12)
                      n114 = Build Array (concatenate)(w138, w137) -> (w135:string[])
                      n115 = Build Array (concatenate)(w140, w136) -> (w139:string[])
                      n116 = local write "Temp Headers"(w135) -> ()
                      n117 = local write "Temp Values"(w139) -> ()
                    }
                    frame #3 {
                      w149 = 2.0  # # of interfaces
                      w154 = 16.0217656  # Unit Conversion
                      n118 = local read "Temp # of atoms"() -> (w156:i32)
                      n119 = local read "OSZICAR Raw Array"() -> (w163:T7)
                      n120 = local read "Temp Headers"() -> (w160:string[])
                      n121 = Build Path(base path=w166, name or relative path="OSZICAR") -> (appended path=w165:path)
                      n122 = call "Parse OSZICAR (Energies).vi"("# of Atoms"=w156, "OSZICAR File"=w165) -> ("Summary Values"=w157:string[], "Summary Headers"=w158:string[], "OSZICAR Raw"=w164:T16, "Extracted Parameters"=w153:T17)  [unwired: 6 in]
                      n123 = Unbundle By Name(w153) -> ("Total Formation Energy (eV)"=w152:dbl)
                      n124 = Build Array (concatenate)(w160, w158, "Interfacial Energy (J/m²)") -> (w159:string[])
                      n125 = Build Array (concatenate)(w163, w164) -> (→"OSZICAR Raw Array":T7)
                      n126 = local read "Temp Interfacial Area"() -> (w151:dbl)
                      n127 = local write "Temp Headers"(w159) -> ()
                      n128 = Divide(x=w152, y=w151) -> (x/y=w155:dbl)
                      n129 = Multiply(x=w154, y=w155) -> (x*y=w150:dbl)
                      n130 = Divide(x=w150, y=w149) -> (x/y=w148:dbl)
                      n131 = local read "Temp Values"() -> (w162:string[])
                      n132 = Number To Fractional String(number=w148) -> (F-format string=w147:string)  [unwired: 3 in]
                      n133 = Build Array (concatenate)(w162, w157, w147) -> (w161:string[])
                      n134 = local write "Temp Values"(w161) -> ()
                    }
                    frame #4 {
                      n135 = local read "Temp Headers"() -> (w174:string[])
                      n136 = Build Path(base path=w176, name or relative path="OUTCAR") -> (appended path=w177:path)
                      n137 = call "Parse OUTCAR.vi"("OUTCAR File"=w177) -> ("error out"=w168:errorcluster, "Calc Time (Hrs)"=w171:dbl)  [unwired: 8 in, 1 out]
                      n138 = local read "Temp Values"() -> (w172:string[])
                      n139 = Build Array (concatenate)(w174, "Calc Time (hrs)") -> (w175:string[])
                      n140 = Number To Fractional String(number=w171) -> (F-format string=w169:string)  [unwired: 3 in]
                      n141 = local write "Temp Headers"(w175) -> ()
                      n142 = Build Array (concatenate)(w172, w169) -> (w173:string[])
                      n143 = local write "Temp Values"(w173) -> ()
                    }
                    frame #5 {
                      n144 = case shown="True" "Load DOS" {
                        tunnel: w179 -> [_ w189]
                        tunnel: [_ w188] -> _
                        tunnel: [_ w184] -> w182
                        frame False {
                        }
                        frame True {
                          n145 = Build Path(base path=w189, name or relative path="DOSCAR") -> (appended path=w191:path)
                          n146 = call "Parse DOSCAR.vi"("Only total DOS"="Only total DOS", "Path"=w191) -> ("error out"=w188:errorcluster, "Atomic-decomposed DOS"=w185:T18, "Total DOS"=w186:T19, "DOS Summary"=w187:T20)  [unwired: 6 in]
                          n147 = Bundle("DOS Summary"=w187, "Total DOS"=w186, "Atomic-decomposed DOS"=w185) -> (w184:T21)  [unwired: 1 in]
                        }
                      }
                      n148 = local read "DOS Array"() -> (w180:T4)
                      n149 = Build Array (concatenate)(w180, w182) -> (→"DOS Array":T14)
                    }
                    frame #6 {
                      n150 = Build Path(base path=w199, name or relative path="README.txt") -> (appended path=w201:path)
                      n151 = call <vilib>:"Check if File or Folder Exists.vi"("path"=w201) -> ("file or folder exists?"=w200:bool)  [unwired: 8 in, 2 out]
                      n152 = case shown="True" w200 {
                        tunnel: w201 -> [_ w207]
                        tunnel: [_ w204] -> w194
                        tunnel: [_ w203] -> w193
                        frame False {
                        }
                        frame True {
                          n153 = call-poly <vilib>:"Read From Spreadsheet File.vi"("file path (dialog if empty)"=w207) -> ("all rows"=w206:string[][])  [unwired: 6 in, 4 out]
                          n154 = Index Array(array=w206, index (col) #1=0 ("disabled index (col)")) -> (element #1=w204:string[], element #2=w203:string[])  [unwired: 3 in]
                        }
                      }
                      n155 = local read "Temp Headers"() -> (w197:string[])
                      n156 = local read "Temp Values"() -> (w195:string[])
                      n157 = Build Array (concatenate)(w197, w194) -> (w198:string[])
                      n158 = Build Array (concatenate)(w195, w193) -> (w196:string[])
                      n159 = local write "Temp Headers"(w198) -> ()
                      n160 = local write "Temp Values"(w196) -> ()
                    }
                    frame #7 {
                      n161 = local read "All DFT Data Summary"() -> (w211:T8)
                      n162 = Unbundle By Name(w211) -> ("Headers"=w221:string[], "Relaxation Data"=w214:string[][])
                      n163 = local read "Temp Headers"() -> (w219:string[])
                      n164 = local read "Temp Values"() -> (w218:string[])
                      n165 = Index Array(array=w214, index (row)=w213) -> (element=w220:string[])  [unwired: 1 in]
                      n166 = call "Updated Dynamic Headers.vi"("Old Data"=w220, "New Data"=w218, "This Data's Headers"=w219, "Old Headers"=w221) -> ("Formatted New Data"=w209:string[], "Merged Headers"=w210:string[])  [unwired: 6 in]
                      n167 = Build Array (concatenate)(w209, w214) -> (w217:string[][])
                      n168 = Delete From Array(array=w217, index (row)=0) -> (array with subset deleted=w215:string[][])  [unwired: 2 in, 1 out]
                      n169 = Replace Array Subset(array=w215, new element=w209, index (row)=w213) -> (w212:string[][])  [unwired: 1 in]
                      n170 = Bundle By Name(cluster=w211, "Headers"=w210, "Relaxation Data"=w212) -> (→"All DFT Data Summary":T8)
                    }
                  }
                }
                frame True {
                  n171 = local read "Vasp DB UDL"() -> (w226:path)
                  n172 = call-poly <vilib>:"DB Tools Open Connection.vi"("connection information"=w226) -> ("connection reference"=w227:T22)  [unwired: 7 in, 1 out]
                  n173 = stacked-sequence {
                    tunnel: w227 -> [_ w233 _ w267 w308 w312 _]
                    tunnel: w225 -> [w228 w232 _ w261 _ _ _]
                    tunnel: [_ _ w252 _ _ _ _] -> w224
                    tunnel: [_ _ w251 _ _ _ _] -> w223
                    tunnel: w222 -> [_ w231 w250 _ _ _ _]
                    frame #0 {
                      n174 = local read "Loaded DFT Paths"() -> (w230:path[])
                      n175 = Build Array (concatenate)(w230, w228) -> (w229:path[])
                      n176 = local write "Loaded DFT Paths"(w229) -> ()
                    }
                    frame #1 {
                      # "No need to update"
                      n177 = disable-structure shown="Disabled" {
                        disable-tunnel: w233 -> [w249 _]
                        disable-tunnel: w232 -> [w248 _]
                        disable-tunnel: [w243 _] -> _
                        disable-tunnel: [w242 _] -> _
                        disable-tunnel: w231 -> [w237 _]
                        frame Disabled {
                          n178 = local read "All DFT Data Summary"() -> (w240:T8)
                          n179 = Unbundle By Name(w240) -> ("Headers"=w241:string[], "Relaxation Data"=w235:string[][])
                          n180 = call "Query Headers and Data from VASP DB.vi"("Full Path"=w248, "connection reference"=w249) -> ("Data"=w242:string[], "Headers"=w243:string[])  [unwired: 6 in, 2 out]
                          n181 = Index Array(array=w235, index (row)=w237) -> (element=w236:string[])  [unwired: 1 in]
                          n182 = call "Updated Dynamic Headers.vi"("Old Data"=w236, "New Data"=w242, "This Data's Headers"=w243, "Old Headers"=w241) -> ("Formatted New Data"=w244:string[], "Merged Headers"=w239:string[])  [unwired: 6 in]
                          n183 = Build Array (concatenate)(w235, w244) -> (w247:string[][])
                          n184 = Delete From Array(array=w247, index (row)=0) -> (array with subset deleted=w245:string[][])  [unwired: 2 in, 1 out]
                          n185 = Replace Array Subset(array=w245, new element=w244) -> (w234:string[][])  [unwired: 2 in]
                          n186 = Bundle By Name(cluster=w240, "Headers"=w239, "Relaxation Data"=w234) -> (w238:T8)
                          n187 = local write "All DFT Data Summary"(w238) -> ()
                        }
                        frame Enabled {
                        }
                      }
                    }
                    frame #2 {
                      n188 = local read "All DFT Data Summary"() -> (w254:T8)
                      n189 = Unbundle By Name(w254) -> ("Headers"=w252:string[], "Relaxation Data"=w253:string[][])
                      n190 = Index Array(array=w253, index (row)=w250) -> (element=w251:string[])  [unwired: 1 in]
                    }
                    frame #3 {
                      n191 = Path To String(path=w261) -> (string=w260:string)
                      n192 = Concatenate Strings("WHERE Full_Directory ='", w260, "'" ("string")) -> (w262:string)
                      n193 = call <vilib>:"DB Tools Select Data.vi"("condition"=w262, "columns"=string[] ["CONTCAR_Structure_ID", "OSZICAR_ID", "DOSCAR_ID"], "table"="DFT_Summary", "connection reference"=w267) -> ("data"=w259:variant[][])  [unwired: 2 in, 2 out]
                      n194 = Index Array(array=w259, index (row)=0) -> (element=w257:variant[])  [unwired: 1 in]
                      n195 = for {
                        tunnel: w257 -> [w270] mode=indexing
                        tunnel: [w268] -> w256 mode=indexing
                        n196 = xnode "Database Variant To Data"("database variant"=w270, "type"="") -> ("data"=w268:string)  [unwired: 1 in, 1 out]
                      }
                      n197 = Array To Cluster(array=w256) -> (cluster=→"IDs":T23)
                    }
                    frame #4 {
                      n198 = local read "IDs"() -> (w306:T2)
                      n199 = Unbundle By Name(w306) -> ("CONTCAR ID"=w305:string)
                      n200 = call "Import Structure from DB.vi"("Structure ID"=w305, "connection reference"=w308) -> ("Loaded Structure"=w304:T5)  [unwired: 7 in, 2 out]
                      n201 = local read "Structures"() -> (w309:T12)
                      n202 = Unbundle By Name(w304) -> ("# of atoms"=w303:i32)
                      n203 = Build Array (concatenate)(w309, w304) -> (w307:T12)
                      n204 = local write "Temp # of atoms"(w303) -> ()
                      n205 = local write "Structures"(w307) -> ()
                    }
                    frame #5 {
                      n206 = local read "IDs"() -> (w315:T2)
                      n207 = local read "Temp # of atoms"() -> (w314:i32)
                      n208 = Unbundle By Name(w315) -> ("OSZICAR ID"=w313:string)
                      n209 = local read "OSZICAR Raw Array"() -> (w316:T7)
                      n210 = call "Import Energies (OSZICAR) from DB.vi"("# of Atoms"=w314, "OSZICAR ID"=w313, "connection reference"=w312) -> ("OSZICAR Raw"=w311:T16)  [unwired: 5 in, 3 out]
                      n211 = Build Array (concatenate)(w316, w311) -> (w310:T7)
                      n212 = local write "OSZICAR Raw Array"(w310) -> ()
                    }
                    frame #6 {
                      n213 = disable-structure shown="Disabled" {
                        frame Disabled {
                          n214 = local read "DOS Array"() -> (w318:T4)
                          n215 = local read "IDs"() -> (w317:T2)
                          n216 = local read "Only total DOS"() -> ()  [unwired: 1 out]
                          n217 = Unbundle By Name(w317) -> ()  [unwired: 1 out]
                          n218 = Build Array (concatenate)(w318) -> ()  [unwired: 1 in, 1 out]
                        }
                        frame Enabled {
                        }
                      }
                    }
                  }
                }
              }
            }
          }
        }
        n219 = call <vilib>:"Set Busy.vi"() -> ("error out"=w88:errorcluster)  [unwired: 10 in, 1 out]
        n220 = property on="Bivariate Y-Axis" class="CmbBox"("Strings[]"=w87) -> ()  [unwired: 2 in, 2 out]
        n221 = property on="Grouping Col List" class="Ring (strict)"("Strings []"=w87) -> ()  [unwired: 2 in, 2 out]
        n222 = property on="Bivariate X-Axis" class="CmbBox"("Strings[]"=w87) -> ()  [unwired: 2 in, 2 out]
        n223 = property on="Parameter Analysis Y-Axis" class="Ring (strict)"("Strings []"=w87) -> ()  [unwired: 2 in, 2 out]
        n224 = property on="Details" class="MCListbox (strict)"(error in=w88, "ColHdrString"=w87, "ItemNames"=w86) -> (error out=w89:errorcluster)  [unwired: 1 in, 1 out]
        n225 = case shown="\"Interfacial Energy\"" "Tab Control" {
          tunnel: w89 -> [_ _ _ _ _ _ _ _ _]
          frame "Overview", Default {
            n226 = property on="Plot Relaxation" class="Bool (strict)"("Val(Sgnl)"=TRUE ("Value (Signaling)")) -> ()  [unwired: 2 in, 2 out]
            n227 = property on="Plot DOS" class="Bool (strict)"("Val(Sgnl)"=TRUE ("Value (Signaling)")) -> ()  [unwired: 2 in, 2 out]
            n228 = property on="Plot Variability" class="Bool (strict)"("Val(Sgnl)"=TRUE ("Value (Signaling)")) -> ()  [unwired: 2 in, 2 out]
          }
          frame "Relaxation" {
            n229 = property on="Plot Relaxation" class="Bool (strict)"("Val(Sgnl)"=TRUE ("Value (Signaling)")) -> ()  [unwired: 2 in, 2 out]
          }
          frame "Structure" {
            n230 = property on="Plot Structures" class="Bool (strict)"("Val(Sgnl)"=TRUE ("Value (Signaling)")) -> ()  [unwired: 2 in, 2 out]
          }
          frame "DOS" {
            n231 = property on="Plot DOS" class="Bool (strict)"("Val(Sgnl)"=TRUE ("Value (Signaling)")) -> ()  [unwired: 2 in, 2 out]
          }
          frame "Variability" {
            n232 = property on="Plot Variability" class="Bool (strict)"("Val(Sgnl)"=TRUE ("Value (Signaling)")) -> ()  [unwired: 2 in, 2 out]
          }
          frame "Bivariate" {
            n233 = property on="Plot Bivariate" class="Bool (strict)"("Val(Sgnl)"=TRUE ("Value (Signaling)")) -> ()  [unwired: 2 in, 2 out]
          }
          frame "Band Edge Diagram" {
            n234 = property on="Plot Band Edge Diagram" class="Bool (strict)"("Val(Sgnl)"=TRUE ("Value (Signaling)")) -> ()  [unwired: 2 in, 2 out]
          }
          frame "Defect Formation Energy" {
            n235 = property on="Plot Formation Energy" class="Bool (strict)"("Val(Sgnl)"=TRUE ("Value (Signaling)")) -> ()  [unwired: 2 in, 2 out]
          }
          frame "Interfacial Energy" {
            n236 = local read "GB Size Factor"() -> (w329:dbl)
            n237 = property on="GB Size Factor" class="DigNum (strict)"("Val(Sgnl)"=w329) -> ()  [unwired: 2 in, 2 out]
          }
        }
        n238 = call <vilib>:"Unset Busy.vi"("error in (no error)"=w89) -> ()  [unwired: 10 in, 1 out]
      }
      event "Plot Relaxation": Value Change {
        n239 = event-data() -> ()  [unwired: 1 in, 5 out]
        n240 = local read "All DFT Data Summary"() -> (w331:T8)
        n241 = Unbundle By Name(w331) -> ("Relaxation Data"=w330:string[][])
        n242 = local read "Selection List"() -> (w337:i32[])
        n243 = for {
          tunnel: w337 -> [w365] mode=indexing
          tunnel: [w361] -> w334 mode=indexing
          tunnel: [w366] -> w332 mode=indexing
          tunnel: w330 -> [w357]
          n244 = Index Array(array=w357, index (row)=w365) -> (element=w364:string[])  [unwired: 1 in]
          n245 = local read "Loaded DFT Paths"() -> (w356:path[])
          n246 = Index Array(array=w364, index #2=2 ("index"), index #3=3 ("index")) -> (element #1=w363:string, element #2=w361:string, element #3=w359:string)  [unwired: 1 in]
          n247 = local read "OSZICAR Raw Array"() -> (w353:T7)
          n248 = String To Path(string=w363) -> (path=w355:path)
          n249 = Decimal String To Number(string=w359) -> (number=w358:i32)  [unwired: 2 in, 1 out]
          n250 = Search 1D Array(1D array=w356, element=w355) -> (index of element=w354:i32)  [unwired: 1 in]
          n251 = Index Array(array=w353, index=w354) -> (element=w352:T16)
          n252 = case shown="\"Formation Energy/Atom\"" "Relaxation Y-Axis" {
            tunnel: w352 -> [w370 w372 w376 w380]
            tunnel: [w369 w373 w377 w379] -> w367
            tunnel: w358 -> [_ w374 w378 _]
            frame "Energy", Default {
              n253 = Unbundle By Name(w370) -> ("Ionic Relaxation Energies Array (eV)"=w369:dbl[])
            }
            frame "Energy/Atom" {
              n254 = Unbundle By Name(w372) -> ("Ionic Relaxation Energies Array (eV)"=w371:dbl[])
              n255 = Divide(x=w371, y=w374) -> (x/y=w373:dbl[])
            }
            frame "Formation Energy/Atom" {
              n256 = Unbundle By Name(w376) -> ("Bulk Formation Energies Array (eV)"=w375:dbl[])
              n257 = Divide(x=w375, y=w378) -> (x/y=w377:dbl[])
            }
            frame "Formation Energy" {
              n258 = Unbundle By Name(w380) -> ("Bulk Formation Energies Array (eV)"=w379:dbl[])
            }
          }
          n259 = Bundle("Bulk Formation Energies Array (eV)"=w367) -> (w366:T24)  [unwired: 1 in]
        }
        "Relaxation" <- w332
        "Overview - Relaxation" <- w332
        n260 = Array Size(array=w334) -> (size(s)=w333:i32)
        n261 = local read "Color Array Type"() -> (w336:T11)
        n262 = call "Num of Colors to Color Array.vi"("# of Colors"=w333, "Color Array Type"=w336) -> ("Colors Array"=w335:u32[])  [unwired: 3 in]
        n263 = for {
          N -> [w343]
          tunnel: w334 -> [w342] mode=indexing
          tunnel: w335 -> [w341] mode=indexing
          i -> [w344]
          n264 = control-ref of="Relaxation"() -> (w339:refnum<vi>)
          n265 = control-ref of="Overview - Relaxation"() -> (w340:refnum<vi>)
          n266 = Build Array(w339, w340) -> (w338:refnum<vi>[])
          n267 = for {
            tunnel: w344 -> [w351]
            tunnel: w343 -> [w350]
            tunnel: w342 -> [w349]
            tunnel: w341 -> [w347]
            tunnel: w338 -> [w345] mode=indexing
            n268 = property on="Property Node" class="WFGraph (strict)"(reference=w345, "Active Plot"=w351, "LegNumRows"=w350, "Plot.Plot Name"=w349, "Plot.Point Style"=u8 2, "Plot.Fill/Pt. Color"=w347, "Plot.Plot Interpolation"=u8 0) -> ()  [unwired: 1 in, 2 out]
          }
        }
      }
      event "Relaxation Y-Axis": Value Change {
        n269 = event-data() -> ("NewVal"=w381:string)  [unwired: 1 in, 4 out]
        n270 = property on="Relaxation" class="WFGraph (strict)"("YScale.NameLbl.Text"=w381) -> ()  [unwired: 2 in, 2 out]
        n271 = property on="Overview - Relaxation" class="WFGraph (strict)"("YScale.NameLbl.Text"=w381) -> ()  [unwired: 2 in, 2 out]
        n272 = property on="Plot Relaxation" class="Bool (strict)"("Val(Sgnl)"=TRUE ("Value (Signaling)")) -> ()  [unwired: 2 in, 2 out]
      }
      event "Tab Control": Value Change {
        n273 = event-data() -> ("NewVal"=w383:T9)  [unwired: 1 in, 4 out]
        n274 = case shown="\"Overview\", Default" w383 {
          frame "Overview", Default {
            (unwired) 0 ("Value (Signaling)")
            n275 = property on="Plot Relaxation" class="Bool (strict)"("Val(Sgnl)"=TRUE ("Value (Signaling)")) -> ()  [unwired: 2 in, 2 out]
            n276 = property on="Plot Variability" class="Bool (strict)"("Val(Sgnl)"=TRUE ("Value (Signaling)")) -> ()  [unwired: 2 in, 2 out]
            n277 = property on="Plot DOS" class="Bool (strict)"("Val(Sgnl)"=TRUE ("Value (Signaling)")) -> ()  [unwired: 2 in, 2 out]
          }
          frame "Relaxation" {
            n278 = property on="Plot Relaxation" class="Bool (strict)"("Val(Sgnl)"=TRUE ("Value (Signaling)")) -> ()  [unwired: 2 in, 2 out]
          }
          frame "Structure" {
            n279 = property on="Plot Structures" class="Bool (strict)"("Val(Sgnl)"=TRUE ("Value (Signaling)")) -> ()  [unwired: 2 in, 2 out]
          }
          frame "DOS" {
            n280 = property on="Plot DOS" class="Bool (strict)"("Val(Sgnl)"=TRUE ("Value (Signaling)")) -> ()  [unwired: 2 in, 2 out]
          }
          frame "Variability" {
            n281 = property on="Plot Variability" class="Bool (strict)"("Val(Sgnl)"=TRUE ("Value (Signaling)")) -> ()  [unwired: 2 in, 2 out]
          }
          frame "Bivariate" {
            n282 = property on="Plot Bivariate" class="Bool (strict)"("Val(Sgnl)"=TRUE ("Value (Signaling)")) -> ()  [unwired: 2 in, 2 out]
          }
          frame "Defect Formation Energy" {
            n283 = property on="Plot Formation Energy" class="Bool (strict)"("Val(Sgnl)"=TRUE ("Value (Signaling)")) -> ()  [unwired: 2 in, 2 out]
          }
        }
      }
      event "Plot DOS", "Always Show Bulk": Value Change {
        n284 = event-data() -> ()  [unwired: 1 in, 5 out]
        n285 = local read "All DFT Data Summary"() -> (w414:T8)
        n286 = local read "Selection List"() -> (w411:i32[])
        n287 = Unbundle By Name(w414) -> ("Relaxation Data"=w413:string[][])
        n288 = Index Array(array=w411) -> (element=w410:i32)  [unwired: 1 in]
        n289 = Index Array(array=w413, index (row)=w410) -> (element=w409:string[])  [unwired: 1 in]
        n290 = local read "Loaded DFT Paths"() -> (w406:path[])
        n291 = Index Array(array=w409, index #2=2 ("index")) -> (element #1=w408:string, element #2=w399:string)  [unwired: 1 in]
        n292 = String To Path(string=w408) -> (path=w405:path)
        n293 = Build Array (concatenate)(w399, "Total DOS" ("element"), string[] ["", "", "", "", "", "", ""] ("appended array")) -> (w398:string[])
        n294 = local read "DOS Array"() -> (w404:T4)
        n295 = local read "Structures"() -> (w403:T12)
        n296 = Search 1D Array(1D array=w406, element=w405) -> (index of element=w402:i32)  [unwired: 1 in]
        n297 = Index Array(array=w403, index=w402) -> (element=w401:T5)
        n298 = Index Array(array=w404, index=w402) -> (element=→"Selected DOS":T3)
        n299 = Unbundle By Name(w401) -> ("Atoms Array"=w400:T25)
        n300 = Build Array(w398) -> (w396:string[][])
        n301 = for {
          tunnel: w400 -> [w423] mode=indexing
          shift-right: [w419] -> w412
          shift-left: w396 -> [w418]
          tunnel: w399 -> [w417]
          n302 = Unbundle By Name(w423) -> ("Atom Name"=w420:string, "Positions (Direct)"=w422:dbl[][], "Positions (Cartesian)"=w421:dbl[][])
          n303 = for {
            tunnel: w422 -> [w432] mode=indexing
            tunnel: w421 -> [w431] mode=indexing
            tunnel: w420 -> [w430]
            shift-right: [w426] -> w419
            shift-left: w418 -> [w425]
            tunnel: w417 -> [w424]
            n304 = Number To Fractional String(number=w432) -> (F-format string=w429:string[])  [unwired: 3 in]
            n305 = Number To Fractional String(number=w431) -> (F-format string=w428:string[])  [unwired: 3 in]
            n306 = Build Array (concatenate)(w424, w430, w429, w428) -> (w427:string[])
            n307 = Build Array (concatenate)(w425, w427) -> (w426:string[][])
          }
        }
        n308 = property on="DOS Options" class="MCListbox (strict)"("ItemNames"=w412) -> (error out=w394:errorcluster)  [unwired: 2 in, 1 out]
        n309 = disable-structure shown="Disabled" {
          disable-tunnel: w394 -> [w415 _]
          frame Disabled {
            n310 = property on="DOS Options" class="MCListbox (strict)"(error in=w415, "Val(Sgnl)"=i32[] [0] ("Value (Signaling)")) -> ()  [unwired: 1 in, 2 out]
          }
          frame Enabled {
          }
        }
      }
      event "DOS Options": Value Change {
        n311 = event-data() -> ()  [unwired: 1 in, 5 out]
        n312 = local read "Selected DOS"() -> (w436:T3)
        n313 = Unbundle By Name(w436) -> ("DOS Summary.Fermi Level (eV)"=w439:dbl, "DOS Summary.# Filled States"=w434:dbl)
        n314 = Unbundle By Name(w436) -> ("Total DOS.Energy (eV)"=w438:dbl[])
        n315 = Subtract(x=w438, y=w439) -> (x-y=w437:dbl[])
        n316 = Array Size(array=w438) -> (size(s)=w440:i32)
        n317 = Initialize Array(0.0 ("Numeric"), w440) -> (w448:dbl[])
        n318 = for {
          tunnel: "DOS Options" -> [w462] mode=indexing
          shift-right: [w459] -> w435
          shift-left: w448 -> [w460]
          tunnel: w436 -> [w461]
          n319 = case shown="0" w462 {
            selector: w462 -> [_ w476]
            tunnel: w461 -> [w464 w478]
            tunnel: w460 -> [_ w468]
            tunnel: [w463 w465] -> w459
            frame 0 {
              n320 = Unbundle By Name(w464) -> ("Total DOS.Total DOS"=w463:dbl[])
            }
            frame 1, Default {
              n321 = Unbundle By Name(w478) -> ("Atomic-decomposed DOS"=w477:T18)
              n322 = Decrement(x=w476) -> (x-1=w475:i32)
              n323 = Index Array(array=w477, index=w475) -> (element=w474:T26)
              n324 = Build Array(FALSE ("element"), "S Orbitals", "P Orbital", "P Orbital", "P Orbital", "D Orbitals", "D Orbitals", "D Orbitals", "D Orbitals", "D Orbitals") -> (w469:bool[])
              n325 = Unbundle By Name(w474) -> ("DOS"=w473:dbl[][])
              n326 = Transpose 2D Array(2D array=w473) -> (transposed array=w472:dbl[][])
              n327 = for {
                shift-right: [w480] -> w465
                shift-left: w468 -> [w479]
                tunnel: w472 -> [w482] mode=indexing
                tunnel: w469 -> [w481] mode=indexing
                n328 = case shown="False" w481 {
                  tunnel: w482 -> [_ w486]
                  tunnel: [w483 w485] -> w480
                  tunnel: w479 -> [w483 w484]
                  frame False {
                  }
                  frame True {
                    n329 = Add(x=w486, y=w484) -> (x+y=w485:dbl[])
                  }
                }
              }
            }
          }
        }
        n330 = local read "DOS Plot Names"() -> (w445:string[])
        n331 = Build Array (concatenate)("Current", w445) -> (w443:string[])
        n332 = Array Size(array=w443) -> (size(s)=w458:i32)
        n333 = call "Num of Colors to Color Array.vi"("# of Colors"=w458, "Color Array Type"="Color Array Type") -> ("Colors Array"=w455:u32[])  [unwired: 3 in]
        n334 = Divide(x=w435, y=w434) -> (x/y=w433:dbl[])
        n335 = Bundle(w437, w433) -> (w447:cluster{dbl[], dbl[]})  [unwired: 1 in]
        n336 = case shown="True" "Always Show Bulk" {
          tunnel: [w487 w500] -> w446
          tunnel: [w489 w498] -> w452
          tunnel: w455 -> [w490 w496]
          tunnel: [w490 w495] -> w453
          tunnel: w443 -> [w489 w493]
          tunnel: w447 -> [w488 w492]
          frame False {
            n337 = Build Array(w488) -> (w487:cluster{dbl[], dbl[]}[])
          }
          frame True {
            n338 = Build Array (concatenate)("Bulk", w493) -> (w498:string[])
            n339 = Build Array(cluster{dbl[], dbl[]} {array[2000 elements], array[2000 elements]}, w492) -> (w500:cluster{dbl[], dbl[]}[])
            n340 = Build Array (concatenate)(u32 16777222 ("Color Box"), u32 11776947 ("Color Box"), w496) -> (w495:u32[])
          }
        }
        n341 = local read "Saved DOS Plots"() -> (w442:cluster{dbl[], dbl[]}[])
        n342 = control-ref of="DOS PLot"() -> (w454:refnum<vi>)
        n343 = Build Array (concatenate)(w446, w442) -> (→"DOS PLot" →"Overview DOS PLot":cluster{dbl[], dbl[]}[])
        n344 = call "Format XY Plot.vi"("Plot Interpolation"=u8 2, "Colors Array"=w453, "Plot Names"=w452, "XY Graph Reference"=w454) -> ()  [unwired: 8 in]
      }
      event "S Orbitals", "P Orbital", "D Orbitals": Value Change {
        n345 = event-data() -> ()  [unwired: 1 in, 5 out]
        n346 = local read "DOS Options"() -> (w501:i32[])
        n347 = property on="DOS Options" class="MCListbox (strict)"("Val(Sgnl)"=w501) -> ()  [unwired: 2 in, 2 out]
      }
      event "DOS Sum and Plot": Value Change {
        n348 = event-data() -> ()  [unwired: 1 in, 5 out]
        n349 = local read "DOS PLot"() -> (w509:cluster{dbl[], dbl[]}[])
        n350 = local read "DOS Plot Names"() -> (w503:string[])
        n351 = local read "DOS Options"() -> (w502:i32[])
        n352 = local read "Saved DOS Plots"() -> (w506:cluster{dbl[], dbl[]}[])
        n353 = Index Array(array=w509) -> (element=w508:cluster{dbl[], dbl[]})  [unwired: 1 in]
        n354 = property on="DOS Options" class="MCListbox (strict)"("Val(Sgnl)"=w502) -> ()  [unwired: 2 in, 2 out]
        n355 = Build Array (concatenate)(w503, "Plot Name") -> (→"DOS Plot Names":string[])
        n356 = Build Array (concatenate)(w506, w508) -> (→"Saved DOS Plots":cluster{dbl[], dbl[]}[])
      }
      event "Erase": Value Change {
        w511 = cluster{dbl[], dbl[]}[] [] ("DOS PLot")
        n357 = event-data() -> ()  [unwired: 1 in, 5 out]
        n358 = local write "DOS Plot Names"(string[] [] ("DOS Plot Names")) -> ()
        n359 = local write "DOS PLot"(w511) -> ()
        n360 = local write "Saved DOS Plots"(w511) -> ()
      }
      event "Plot Band Edge Diagram", "Low Density Cutoff", "Step or #pts", "Style": Value Change {
        n361 = event-data() -> ()  [unwired: 1 in, 5 out]
        n362 = local read "All DFT Data Summary"() -> (w515:T8)
        n363 = Unbundle By Name(w515) -> ("Relaxation Data"=w514:string[][])
        n364 = local read "Selection List"() -> (w516:i32[])
        n365 = for {
          tunnel: w516 -> [w529] mode=indexing
          tunnel: w514 -> [w530]
          shift-right: [w519] -> w513
          shift-left: cluster{"Array":dbl[], dbl[]}[] [] -> [w518]
          n366 = Index Array(array=w530, index (row)=w529) -> (element=w528:string[])  [unwired: 1 in]
          n367 = local read "Loaded DFT Paths"() -> (w532:path[])
          n368 = Index Array(array=w528, index #2=2 ("index")) -> (element #1=w534:string)  [unwired: 1 in, 1 out]
          n369 = String To Path(string=w534) -> (path=w531:path)
          n370 = local read "DOS Array"() -> (w527:T4)
          n371 = Search 1D Array(1D array=w532, element=w531) -> (index of element=w525:i32)  [unwired: 1 in]
          n372 = local read "Structures"() -> (w526:T12)
          n373 = Index Array(array=w527, index=w525) -> (element=w517:T3)
          n374 = Unbundle By Name(w517) -> ()  [unwired: 1 out]
          n375 = Index Array(array=w526, index=w525) -> (element=w524:T5)
          n376 = call "Extract Band Diagram from Atoms and DOS.vi"("Low Density Cutoff"="Low Density Cutoff", "Style"="Style", "Step or #pts"="Step or #pts", "Structure"=w524) -> ("Band Edge Diagram"=w520:cluster{"Array":dbl[], dbl[]}[])  [unwired: 6 in, 1 out]
          n377 = Build Array (concatenate)(w518, w520) -> (w519:cluster{"Array":dbl[], dbl[]}[])
        }
        "Band Edge Diagram" <- w513
      }
      event "Grouping Columns", "Parameter Analysis Y-Axis", "Plot Variability": Value Change {
        n378 = event-data() -> ()  [unwired: 1 in, 5 out]
        n379 = property on="Parameter Analysis Y-Axis" class="Ring (strict)"() -> ("RingText.Text"=w537:string)  [unwired: 2 in, 2 out]
        n380 = property on="Parameter Analysis Graph" class="XYGraph (strict)"("YScale.NameLbl.Text"=w537) -> ()  [unwired: 2 in, 2 out]
        n381 = property on="Overview - Parameter Analysis Graph" class="XYGraph (strict)"("YScale.NameLbl.Text"=w537) -> ()  [unwired: 2 in, 2 out]
        n382 = property on="Details" class="MCListbox (strict)"() -> ("ColHdrString"=w536:string[], "ItemNames"=w535:string[][])  [unwired: 2 in, 2 out]
        n383 = control-ref of="Overview - Parameter Analysis Graph"() -> (w540:refnum<vi>)
        n384 = control-ref of="Parameter Analysis Graph"() -> (w541:refnum<vi>)
        n385 = call "Build Variability Plot from Reference.vi"("Group Cols"="Grouping Columns", "Y-axis Col"="Parameter Analysis Y-Axis", "Column Header Strings"=w536, "Input Table"=w535, "Variability Plot Reference"=w541) -> ()  [unwired: 7 in]
        n386 = call "Build Variability Plot from Reference.vi"("Group Cols"="Grouping Columns", "Y-axis Col"="Parameter Analysis Y-Axis", "Column Header Strings"=w536, "Input Table"=w535, "Variability Plot Reference"=w540) -> ()  [unwired: 7 in]
      }
      event "Plot Bivariate", "Bivariate Y-Axis", "Bivariate X-Axis": Value Change {
        n387 = event-data() -> ()  [unwired: 1 in, 5 out]
        n388 = local read "All DFT Data Summary"() -> (w551:T8)
        n389 = property on="Bivariate Y-Axis" class="CmbBox"() -> ("Strings[]"=w555:string[])  [unwired: 2 in, 2 out]
        n390 = property on="Bivariate X-Axis" class="CmbBox"() -> ("Strings[]"=w553:string[])  [unwired: 2 in, 2 out]
        n391 = property on="Bivariate Plot" class="XYGraph (strict)"("XScale.NameLbl.Text"="Bivariate X-Axis", "YScale.NameLbl.Text"="Bivariate Y-Axis") -> ()  [unwired: 2 in, 2 out]
        n392 = Search 1D Array(1D array=w553, element="Bivariate X-Axis") -> (index of element=w552:i32)  [unwired: 1 in]
        n393 = Search 1D Array(1D array=w555, element="Bivariate Y-Axis") -> (index of element=w554:i32)  [unwired: 1 in]
        n394 = Unbundle By Name(w551) -> ("Relaxation Data"=w550:string[][])
        n395 = local read "Selection List"() -> (w556:i32[])
        n396 = for {
          tunnel: w550 -> [w568]
          tunnel: w556 -> [w564] mode=indexing
          tunnel: w554 -> [w567]
          tunnel: w552 -> [w563]
          tunnel: [w560] -> w547 mode=indexing
          n397 = Index Array(array=w568, index (row) #1=w564, index (col) #1=w563, index (row) #2=w564, index (col) #2=w567) -> (element #1=w566:string, element #2=w565:string)
          n398 = Fract/Exp String To Number(string=w566) -> (number=w562:dbl)  [unwired: 3 in, 1 out]
          n399 = Fract/Exp String To Number(string=w565) -> (number=w561:dbl)  [unwired: 3 in, 1 out]
          n400 = Bundle(w562, w561) -> (w560:cluster{dbl, dbl})  [unwired: 1 in]
        }
        n401 = Sort 1D Array(array=w547) -> (sorted array=w546:cluster{dbl, dbl}[])
        n402 = for {
          tunnel: w546 -> [w559] mode=indexing
          tunnel: [w558] -> w545 mode=indexing
          tunnel: [w557] -> w544 mode=indexing
          n403 = Unbundle(w559) -> (w558:dbl, w557:dbl)
        }
        n404 = Bundle(w545, w544) -> (w543:cluster{dbl[], dbl[]})  [unwired: 1 in]
        n405 = Build Array(w543) -> (→"Bivariate Plot":cluster{dbl[], dbl[]}[])
      }
      event "Bivariate Plot": Shortcut Menu Activation? {
        n406 = event-data() -> ("MenuRef"=w569:refnum<k9>)  [unwired: 1 in, 5 out]
        n407 = Insert Menu Items(8:string[] ["Fit Parabola", "Fit Formula"] ("item names"), 9:w569) -> ()  [unwired: 4 in, 3 out]
        n408 = event-data() -> ()  [unwired: 2 in, 1 out]
      }
      event "Bivariate Plot": Shortcut Menu Selection (User) {
        n409 = event-data() -> ("ItemTag"=w571:string)  [unwired: 1 in, 6 out]
        n410 = case shown="\"Fit Parabola\"" w571 {
          frame Default {
          }
          frame "Fit Parabola" {
            w598 = T27 1 items=["Least Square", "Least Absolute Residual", "Bisquare"] ("method")
            n411 = local read "Bivariate Plot"() -> (w594:cluster{dbl[], dbl[]}[])
            n412 = Index Array(array=w594) -> (element=w593:cluster{dbl[], dbl[]})  [unwired: 1 in]
            n413 = Unbundle(w593) -> (w590:dbl[], w583:dbl[])
            n414 = Array Max & Min(array=w590) -> (max value=w589:dbl, min value=w588:dbl)  [unwired: 2 out]
            n415 = call <vilib>:"General Polynomial Fit.vi"("Y"=w583, "polynomial order"=2, "X"=w590, "method"=w598) -> ("Best Polynomial Fit"=w584:dbl[], "Polynomial Coefficients"=w582:dbl[], "error"=w592:i32)  [unwired: 8 in, 1 out]
            "Polynomial Coefficients" <- w582
            n416 = call <vilib>:"General Error Handler.vi"("[error code] (0)"=w592) -> ()  [unwired: 10 in, 5 out]
            n417 = call "Start and End to Array 2.vi"("Sweep Style"=enum16{"Linear Step", "Linear Pts", "Log Pts"}."Linear Pts", "Step or # Pts"=100.0, "End"=w589, "Start"=w588) -> ("Array"=w591:dbl[])  [unwired: 7 in]
            n418 = call <vilib>:"Goodness of Fit.vi"("Best Fit"=w584, "Y"=w583) -> ("R-square"=w585:dbl)  [unwired: 6 in, 3 out]
            n419 = for {
              tunnel: w591 -> [w606] mode=indexing
              tunnel: w582 -> [w609]
              tunnel: [w602] -> w581 mode=indexing
              n420 = Square(x=w606) -> (x^2=w604:dbl)
              n421 = Index Array(array=w609) -> (element #1=w608:dbl, element #2=w601:dbl, element #3=w605:dbl)  [unwired: 3 in]
              n422 = Multiply(x=w606, y=w601) -> (x*y=w607:dbl)
              n423 = Multiply(x=w605, y=w604) -> (x*y=w603:dbl)
              n424 = Compound Arithmetic op=ADD(w608, w607, w603) -> (w602:dbl)
            }
            n425 = Index Array(array=w582) -> (element #1=w575:dbl, element #2=w572:dbl, element #3=w574:dbl)  [unwired: 3 in]
            n426 = local write "R²"(w585) -> ()
            n427 = Negate(x=w572) -> (-x=w580:dbl)
            n428 = Multiply(x=2.0, y=w574) -> (x*y=w595:dbl)
            n429 = Divide(x=w580, y=w595) -> (x/y=w576:dbl)
            "X_min" <- w576
            n430 = Square(x=w576) -> (x^2=w578:dbl)
            n431 = Bundle("Array"=w591, w581) -> (w600:cluster{"Array":dbl[], dbl[]})  [unwired: 1 in]
            n432 = Multiply(x=w576, y=w572) -> (x*y=w577:dbl)
            n433 = Multiply(x=w574, y=w578) -> (x*y=w579:dbl)
            n434 = Build Array (concatenate)(w594, w600) -> (w599:cluster{"Array":dbl[], dbl[]}[])
            n435 = local write "Bivariate Plot"(w599) -> ()
            n436 = Compound Arithmetic op=ADD(w575, w577, w579) -> (→"Ymin":dbl)
          }
          frame "Fit Formula" {
            n437 = local read "Bivariate Plot"() -> (w618:cluster{dbl[], dbl[]}[])
            n438 = Index Array(array=w618) -> (element=w613:cluster{dbl[], dbl[]})  [unwired: 1 in]
            n439 = Unbundle(w613) -> (w617:dbl[], w612:dbl[])
            n440 = call-poly <vilib>:"Nonlinear Curve Fit.vi"("Y"=w612, "initial parameters"="initial parameters", "X"=w617, "model description"="model description") -> ("best nonlinear fit"=w611:dbl[], "best fit parameters"=→"best fit parameters":dbl[])  [unwired: 7 in, 3 out]
            n441 = Bundle(w617, "best nonlinear fit"=w611) -> (w619:cluster{dbl[], "best nonlinear fit":dbl[]})  [unwired: 1 in]
            n442 = call <vilib>:"Goodness of Fit.vi"("Best Fit"=w611, "Y"=w612) -> ("R-square"=→"R²":dbl)  [unwired: 6 in, 3 out]
            n443 = Build Array (concatenate)(w618, w619) -> (w620:cluster{dbl[], "best nonlinear fit":dbl[]}[])
            n444 = local write "Bivariate Plot"(w620) -> ()
          }
        }
      }
      event "Plot Structures", "Scale", "Auto Setup Camera", "Atom Size": Value Change {
        # "\"Base\" Object is the top level object\nAll atoms are sub-objects of Base"
        n445 = event-data() -> ()  [unwired: 1 in, 5 out]
        n446 = local read "All DFT Data Summary"() -> (w644:T8)
        n447 = local read "Selection List"() -> (w635:i32[])
        n448 = Unbundle By Name(w644) -> ("Relaxation Data"=w643:string[][])
        n449 = Index Array(array=w635) -> (element=w634:i32)  [unwired: 1 in]
        n450 = Index Array(array=w643, index (row)=w634) -> (element=w639:string[])  [unwired: 1 in]
        n451 = local read "Loaded DFT Paths"() -> (w642:path[])
        n452 = Index Array(array=w639, index #2=2 ("index")) -> (element #1=w638:string)  [unwired: 1 in, 1 out]
        n453 = String To Path(string=w638) -> (path=w637:path)
        n454 = local read "Base Object"() -> (w622:refnum<vi>)
        n455 = Search 1D Array(1D array=w642, element=w637) -> (index of element=w633:i32)  [unwired: 1 in]
        n456 = local read "Structures"() -> (w636:T12)
        n457 = Close Reference(reference=w622) -> (error out=w621:errorcluster)  [unwired: 1 in]
        n458 = Index Array(array=w636, index=w633) -> (element=w623:T5)
        "Selected Structure" <- w623
        n459 = Unbundle By Name(w623) -> ("Atoms Array"=w626:T25)
        n460 = call <vilib>:"Create Object.vi"("error in (no error)"=w621, "Name"="Base") -> ("Scene:New Object"=w631:refnum<vi>)  [unwired: 9 out]
        n461 = call "Render Structure.vi"("Options"="Options", "Atom Size"="Atom Size", "Scale"="Scale", "Atomic Structure"=w623, "Base Object"=w631) -> ("Object with atoms"=→"Atomic Structure" →"Base Object":refnum<vi>)  [unwired: 6 in]
        n462 = case shown="True" "Auto Setup Camera" {
          tunnel: w623 -> [_ w667]
          frame False {
          }
          frame True {
            n463 = Unbundle By Name(w667) -> ("Lattice vector a"=w663:dbl[], "Lattice vector b"=w662:dbl[], "Lattice vector c"=w673:dbl[])
            n464 = Negate(x=w663) -> (-x=w661:dbl[])
            n465 = Compound Arithmetic op=ADD(w663, w662, w673) -> (w671:dbl[])
            n466 = local read "Scale"() -> (w670:dbl)
            n467 = Divide(x=w671, y=2.0) -> (x/y=w669:dbl[])
            n468 = Multiply(x=w669, y=w670) -> (x*y=w668:dbl[])
            n469 = Multiply(x=w661, y=2.0 ("Numeric")) -> (x*y=w659:dbl[])
            n470 = Array To Cluster(array=w659) -> (cluster=w664:cluster{"[0]":dbl, "[1]":dbl, "[2]":dbl})
            n471 = Array To Cluster(array=w668) -> (cluster=w666:cluster{"[0]":dbl, "[1]":dbl, "[2]":dbl})
            n472 = Array To Cluster(array=w662) -> (cluster=w665:T28)
            n473 = invoke on="Atomic Structure" class="SceneGraphDisp (strict)" method="Setup Camera"("Camera Position"=w664, "Target"=w666, "Up Direction"=w665) -> ()  [unwired: 3 in, 6 out]
          }
        }
        n474 = for {
          tunnel: w626 -> [w650] mode=indexing
          shift-right: [w646] -> w624
          shift-left: string[][] [] -> [w645]
          n475 = Unbundle By Name(w650) -> ("Atom Name"=w647:string, "Positions (Direct)"=w649:dbl[][], "Positions (Cartesian)"=w648:dbl[][])
          n476 = for {
            tunnel: w649 -> [w658] mode=indexing
            tunnel: w648 -> [w657] mode=indexing
            tunnel: w647 -> [w656]
            shift-right: [w652] -> w646
            shift-left: w645 -> [w651]
            n477 = Number To Fractional String(number=w658) -> (F-format string=w655:string[])  [unwired: 3 in]
            n478 = Number To Fractional String(number=w657) -> (F-format string=w654:string[])  [unwired: 3 in]
            n479 = Build Array (concatenate)(w656, w655, w654) -> (w653:string[])
            n480 = Build Array (concatenate)(w651, w653) -> (w652:string[][])
          }
        }
        n481 = property on="Atom List" class="MCListbox (strict)"("ItemNames"=w624) -> ()  [unwired: 2 in, 2 out]
      }
      event "Atomic Structure": Mouse Down {
        n482 = event-data() -> ("Coords"=w675:T29, "PlatMods"=w676:T30)  [unwired: 1 in, 5 out]
        n483 = property on="Atomic Structure" class="SceneGraphDisp (strict)"() -> ("Position"=w674:T31)  [unwired: 2 in, 2 out]
        n484 = Unbundle By Name(w676) -> ("Ctrl"=w678:bool)
        n485 = Subtract(x=w675, y=w674) -> (x-y=w677:T29)
        n486 = case shown="True" w678 {
          tunnel: w677 -> [_ w681]
          tunnel: w676 -> [_ w682]
          frame False {
          }
          frame True {
            n487 = invoke on="Atomic Structure" class="SceneGraphDisp (strict)" method="PickPoint"("PickPoint"=w681) -> ("PickPoint"=→"PickPoint":T6, "Hit"=w680:bool)  [unwired: 4 in, 3 out]
            n488 = case shown="True" w680 {
              tunnel: w681 -> [_ w684]
              tunnel: w682 -> [_ w688]
              frame False {
              }
              frame True {
                n489 = invoke on="Atomic Structure" class="SceneGraphDisp (strict)" method="Pick Model"("Point"=w684) -> ("Pick Model"=w683:cluster{"Node Path":refnum<vi>[]}[])  [unwired: 3 in, 3 out]
                n490 = Unbundle By Name(w688) -> ("Shift"=w687:bool)
                n491 = Index Array(array=w683) -> (element=w697:cluster{"Node Path":refnum<vi>[]})  [unwired: 1 in]
                n492 = Unbundle By Name(w697) -> ("Node Path"=w695:refnum<vi>[])
                n493 = Array Size(array=w695) -> (size(s)=w696:i32)
                n494 = Decrement(x=w696) -> (x-1=w694:i32)
                n495 = local read "Base Object"() -> (w692:refnum<vi>)
                n496 = Index Array(array=w695, index=w694) -> (element=w693:refnum<vi>)
                n497 = invoke class="SceneObject" method="Object.Object Count"(reference=w692) -> (reference out=w690:refnum<vi>, "Child Count"=w691:i32)  [unwired: 2 in, 1 out]
                n498 = property class="SceneObject"(reference=w693) -> ("Name"=w689:string)  [unwired: 1 in, 2 out]
                n499 = for {
                  N: w691 -> [_]
                  shift-right: [w713] -> _
                  shift-left: w690 -> [w714]
                  tunnel: w689 -> [w709]
                  tunnel: [w708] -> w686
                  i -> [w708]
                  stop <- w711 stop-if-true
                  n500 = invoke class="SceneObject" method="Object.Get Object"(reference=w714, "Child Number"=w708) -> (reference out=w713:refnum<vi>, "Get Child"=w712:refnum<vi>)  [unwired: 2 in, 2 out]
                  n501 = property class="SceneObject"(reference=w712) -> ("Name"=w710:string)  [unwired: 1 in, 2 out]
                  n502 = Equal?(x=w710, y=w709) -> (x = y?=w711:bool)
                }
                n503 = case shown="True" w687 {
                  tunnel: w686 -> [w699 w701]
                  tunnel: [w698 w703] -> w685
                  frame False {
                    n504 = Build Array(w699) -> (w698:i32[])
                  }
                  frame True {
                    n505 = local read "Atom List"() -> (w702:i32[])
                    n506 = Search 1D Array(1D array=w702, element=w701) -> (index of element=w700:i32)  [unwired: 1 in]
                    n507 = case shown="Default" w700 {
                      tunnel: [w704 w707] -> w703
                      tunnel: w702 -> [w704 w706]
                      tunnel: w701 -> [_ w705]
                      frame Default {
                      }
                      frame -1 {
                        n508 = Build Array (concatenate)(w706, w705) -> (w707:i32[])
                      }
                    }
                  }
                }
                n509 = property on="Atom List" class="MCListbox (strict)"("Val(Sgnl)"=w685) -> ()  [unwired: 2 in, 2 out]
              }
            }
          }
        }
      }
      event "Atom List": Value Change {
        n510 = event-data() -> ()  [unwired: 1 in, 5 out]
        n511 = local read "Options"() -> (w715:cluster{"Border?":bool, "Bonds?":bool})
        n512 = local read "Selected Structure"() -> (w719:T5)
        n513 = local read "Atom Size"() -> (w716:dbl)
        n514 = local read "Scale"() -> (w717:dbl)
        n515 = call <vilib>:"Create Object.vi"("Name"="Base") -> ("Scene:New Object"=w720:refnum<vi>)  [unwired: 1 in, 9 out]
        n516 = Multiply(x=w717, y=w716) -> (x*y=w725:dbl)
        n517 = Empty Array?(array="Atom List") -> (empty?=w722:bool)
        n518 = call "Render Structure.vi"("Options"=w715, "Atom Size"=w716, "Scale"=w717, "Atomic Structure"=w719, "Base Object"=w720) -> ("Object with atoms"=w718:refnum<vi>)  [unwired: 6 in]
        n519 = case shown="False" w722 {
          tunnel: "Atom List" -> [w729 _]
          tunnel: w725 -> [w728 _]
          tunnel: [w727 w738] -> w724
          tunnel: w718 -> [w726 w738]
          frame False {
            n520 = for {
              tunnel: w729 -> [w737] mode=indexing
              tunnel: w728 -> [w732]
              tunnel: [w731] -> w727
              tunnel: w726 -> [w730]
              n521 = invoke class="SceneObject" method="Object.Get Object"(reference=w730, "Child Number"=w737) -> (reference out=w731:refnum<vi>, "Get Child"=w736:refnum<vi>)  [unwired: 2 in, 2 out]
              n522 = call <vilib>:"Color Change.vi"("Color"=u32 12961221 ("Highlight Color")) -> ("RGBA"=w734:cluster{"R":sgl, "G":sgl, "B":sgl, "A":sgl})  [unwired: 10 in]
              n523 = call <vilib>:"Create Sphere.vi"("Color"=w734, "Radius"=w732) -> ("New Sphere Refnum"=w735:refnum<vi>)  [unwired: 8 in, 1 out]
              n524 = invoke class="SceneObject" method="Set Drawable"(reference=w736, "Drawable"=w735) -> ()  [unwired: 2 in, 4 out]
            }
          }
          frame True {
          }
        }
        n525 = local write "Atomic Structure"(w724) -> ()
      }
      event "Send to DOS": Value Change {
        n526 = event-data() -> ()  [unwired: 1 in, 5 out]
        n527 = local read "Atom List"() -> (w744:i32[])
        n528 = property on="Plot DOS" class="Bool (strict)"("Val(Sgnl)"=TRUE ("Value (Signaling)")) -> (error out=w741:errorcluster)  [unwired: 2 in, 1 out]
        n529 = Increment(x=w744) -> (x+1=w743:i32[])
        n530 = property on="DOS Options" class="MCListbox (strict)"(error in=w741, "Val(Sgnl)"=w743) -> ()  [unwired: 1 in, 2 out]
        n531 = To Long Integer(number=T15."DOS" ("Tab Control")) -> (32bit integer=w739:i32)
        n532 = local write "Tab Control"(w739) -> ()
      }
      event "Look at Atoms": Value Change {
        n533 = event-data() -> ()  [unwired: 1 in, 5 out]
        n534 = local read "DOS Options"() -> (w748:i32[])
        n535 = To Long Integer(number=T15."Structure" ("Tab Control")) -> (32bit integer=w745:i32)
        n536 = Decrement(x=w748) -> (x-1=w747:i32[])
        n537 = local write "Tab Control"(w745) -> ()
        n538 = property on="Atom List" class="MCListbox (strict)"("Val(Sgnl)"=w747) -> ()  [unwired: 2 in, 2 out]
      }
      event "Animate Relaxation": Value Change {
        n539 = event-data() -> ()  [unwired: 1 in, 5 out]
        n540 = stacked-sequence {
          frame #0 {
            n541 = local read "All DFT Data Summary"() -> (w769:T8)
            n542 = local read "Selection List"() -> (w763:i32[])
            n543 = Unbundle By Name(w769) -> ("Headers"=w755:string[], "Relaxation Data"=w768:string[][])
            n544 = Index Array(array=w763) -> (element=w762:i32)  [unwired: 1 in]
            n545 = local read "Using DB"() -> (w750:bool)
            n546 = Index Array(array=w768, index (row)=w762) -> (element=w766:string[])  [unwired: 1 in]
            n547 = Search 1D Array(1D array=w755, element="DFT_ID") -> (index of element=w753:i32)  [unwired: 1 in]
            n548 = local read "Loaded DFT Paths"() -> (w767:path[])
            n549 = Index Array(array=w766, index #2=w753) -> (element #1=w765:string, element #2=w752:string)  [unwired: 1 in]
            n550 = String To Path(string=w765) -> (path=w749:path)
            n551 = case shown="False" w750 {
              tunnel: w752 -> [_ w791]
              tunnel: [w770 w786] -> w751
              tunnel: w749 -> [w773 _]
              frame False {
                n552 = Build Path(base path=w773, name or relative path="POSCAR") -> (appended path=w771:path)
                n553 = call "Parse POSCAR.vi"("POSCAR File"=w771) -> ("Structure"=w770:T5)  [unwired: 7 in, 3 out]
              }
              frame True {
                w781 = 0 ("index (row)")
                n554 = call <vilib>:"Set Busy.vi"() -> ("error out"=w775:errorcluster)  [unwired: 10 in, 1 out]
                n555 = local read "Vasp DB UDL"() -> (w785:path)
                n556 = call-poly <vilib>:"DB Tools Open Connection.vi"("error in (no error)"=w775, "connection information"=w785) -> ("error out"=w783:errorcluster, "connection reference"=w784:T22)  [unwired: 6 in]
                n557 = Concatenate Strings("WHERE DFT_ID = '" ("condition"), w791, "'" ("string")) -> (w792:string)
                n558 = call <vilib>:"DB Tools Select Data.vi"("condition"=w792, "error in (no error)"=w783, "columns"=string[] ["POSCAR_Structure_ID"], "table"="DFT_Summary", "connection reference"=w784) -> ("error out"=w777:errorcluster, "data"=w782:variant[][], "connection reference out"=w789:T22)  [unwired: 1 in]
                n559 = Index Array(array=w782, index (row)=w781, index (col)=w781) -> (element=w780:variant)
                n560 = xnode "Database Variant To Data"("database variant"=w780, "error in"=w777, "type"="") -> ("data"=w778:string, "error out"=w776:errorcluster)
                n561 = call "Import Structure from DB.vi"("error in (no error)"=w776, "Structure ID"=w778, "connection reference"=w789) -> ("error out"=w774:errorcluster, "Loaded Structure"=w786:T5)  [unwired: 6 in, 1 out]
                n562 = call <vilib>:"Unset Busy.vi"("error in (no error)"=w774) -> ()  [unwired: 10 in, 1 out]
              }
            }
            n563 = Search 1D Array(1D array=w767, element=w749) -> (index of element=w761:i32)  [unwired: 1 in]
            n564 = local read "Structures"() -> (w764:T12)
            n565 = control-ref of="Atomic Structure"() -> (w760:refnum<vi>)
            n566 = Index Array(array=w764, index=w761) -> (element=w759:T5)
            n567 = local read "Scale"() -> (w756:dbl)
            n568 = local read "Atom Size"() -> (w757:dbl)
            n569 = call "Animate two structures.vi"("Atom Size"=w757, "Scale"=w756, "# Frames"="# Frames", "Second Structure"=w751, "First Structure"=w759, "3D Plot Reference"=w760) -> ()  [unwired: 6 in]
          }
        }
      }
      event "Load in VESTA": Value Change {
        n570 = event-data() -> ()  [unwired: 1 in, 5 out]
        n571 = local read "Using DB"() -> (w827:bool)
        n572 = case shown="True" w827 {
          tunnel: [w839 w856] -> w836
          tunnel: [_ w855] -> _
          tunnel: "CONTCAR?" -> [w838 w852]
          frame False {
            n573 = local read "All DFT Data Summary"() -> (w846:T8)
            n574 = local read "Selection List"() -> (w844:i32[])
            n575 = case shown="False" w838 {
              tunnel: ["POSCAR" ("name or relative path") "CONTCAR" ("name or relative path")] -> w837
              frame False {
              }
              frame True {
              }
            }
            n576 = Index Array(array=w844) -> (element=w843:i32)  [unwired: 1 in]
            n577 = Unbundle(w846) -> ("Relaxation Data"=w845:string[][])  [unwired: 1 out]
            n578 = Index Array(array=w845, index (row)=w843, index (col)=0 ("disabled index (col)")) -> (element=w841:string)
            n579 = String To Path(string=w841) -> (path=w840:path)
            n580 = Build Path(base path=w840, name or relative path=w837) -> (appended path=w839:path)
          }
          frame True {
            n581 = local read "All DFT Data Summary"() -> (w873:T8)
            n582 = Unbundle By Name(w873) -> ("Headers"=w863:string[], "Relaxation Data"=w871:string[][])
            n583 = local read "Selection List"() -> (w872:i32[])
            n584 = local read "Vasp DB UDL"() -> (w868:path)
            n585 = Search 1D Array(1D array=w863, element="DFT_ID") -> (index of element=w861:i32)  [unwired: 1 in]
            n586 = Index Array(array=w872) -> (element=w870:i32)  [unwired: 1 in]
            n587 = Index Array(array=w871, index (row)=w870, index (col)=w861) -> (element=w869:string)
            n588 = call-poly <vilib>:"DB Tools Open Connection.vi"("connection information"=w868) -> ("error out"=w864:errorcluster, "connection reference"=w867:T22)  [unwired: 7 in]
            n589 = call "Find Structure ID from DFT ID.vi"("error in (no error)"=w864, "DFT ID"=w869, "connection reference"=w867) -> ("error out"=w874:errorcluster, "POSCAR ID"=w849:string, "CONTCAR_ID"=w850:string, "connection reference out"=w875:T22)  [unwired: 5 in]
            n590 = case shown="False" w852 {
              tunnel: [w879 w880] -> w851
              tunnel: w850 -> [_ w880]
              tunnel: w849 -> [w879 _]
              frame False {
              }
              frame True {
              }
            }
            n591 = call "Import Structure from DB.vi"("error in (no error)"=w874, "Structure ID"=w851, "connection reference"=w875) -> ("error out"=w865:errorcluster, "Loaded Structure"=w878:T5, "connection reference out"=w866:T22)  [unwired: 6 in]
            n592 = Temporary Directory() -> (w859:path)
            n593 = Build Path(base path=w859, name or relative path="OUTCAR") -> (appended path=w858:path)
            n594 = call "Atoms to POSCAR.vi"("Atomic Structure"=w878) -> ("POSCAR File"=w877:string)  [unwired: 10 in]
            n595 = call <vilib>:"DB Tools Close Connection.vi"("error in (no error)"=w865, "connection reference"=w866) -> ("error out"=w854:errorcluster)  [unwired: 5 in]
            n596 = Build Path(base path=w859, name or relative path="CONTCAR") -> (appended path=w856:path)
            n597 = Write to Text File(file (use dialog)=w858, text=" vasp.5.3.3 18Dez12 (build Nov 08 2013 11:21:45) complex                        \n  \n executed on             LinuxIFC date 2014.05.05  14:19:03\n running on   32 total cores\n distrk:  each k-point on   32 cores,    1 groups\n distr:  one band on NCORES_PER_BAND=   8 cores,    4 groups\n\n\n--------------------------------------------------------------------------------------------------------\n\n\n INCAR:\n POTCAR:   PAW_PBE Cd 06Sep2000                   \n POTCAR:  PAW_PBE Te 08Apr2002                    \n POTCAR:   PAW_PBE Cd 06Sep2000    " ("name or relative path"), error in=w854) -> (error out=w857:errorcluster)  [unwired: 1 in, 2 out]
            n598 = Write to Text File(file (use dialog)=w856, text=w877, error in=w857) -> (error out=w855:errorcluster)  [unwired: 1 in, 2 out]
          }
        }
        n599 = Path To String(path="Vesta .exe Location") -> (string=w830:string)
        n600 = Path To String(path=w836) -> (string=w832:string)
        n601 = Concatenate Strings("\"" ("string"), w830, "\" \"" ("string"), w832, "\"" ("string")) -> (w829:string)
        n602 = call <vilib>:"System Exec.vi"("wait until completion? (T)"=FALSE, "command line"=w829) -> ()  [unwired: 6 in, 4 out]
      }
      event "Clean Cache": Value Change {
        n603 = event-data() -> ()  [unwired: 1 in, 5 out]
        n604 = flat-sequence {
          frame #0 {
            n605 = local write "Loaded DFT Paths"(path[] [] ("Loaded DFT Paths")) -> ()
            n606 = local write "OSZICAR Raw Array"(T7 [] ("OSZICAR Raw Array")) -> ()
            n607 = local write "Structures"(T12 [] ("Structures")) -> ()
            n608 = local write "DOS Array"(T14 [] ("DOS Array")) -> ()
            n609 = property on="Selection List" class="MCListbox (strict)"("ItemNames"=string[][] [] ("Item Names")) -> ()  [unwired: 2 in, 2 out]
            n610 = Request Deallocation(TRUE ("flag")) -> ()
          }
        }
      }
      event "Save Summary": Value Change {
        n611 = event-data() -> ()  [unwired: 1 in, 5 out]
        n612 = call "File Dialog"("pattern (all files)"="*.txt") -> ("selected path"=w890:path, "cancelled"=w889:bool, "error out"=w887:errorcluster)  [unwired: 11 in, 1 out]
        n613 = case shown="False" w889 {
          tunnel: w890 -> [w893 _]
          tunnel: w887 -> [_ _]
          frame False {
            n614 = property on="Details" class="MCListbox (strict)"() -> ("ColHdrString"=w892:string[], "ItemNames"=w891:string[][])  [unwired: 2 in, 2 out]
            n615 = Build Array (concatenate)(w892, w891) -> (w894:string[][])
            n616 = call-poly <vilib>:"Write To Spreadsheet File.vi"("2D data"=w894, "file path (dialog if empty)"=w893) -> ()  [unwired: 6 in, 1 out]
          }
          frame True {
          }
        }
      }
      event "Loaded Files", "Plot Formation Energy", "Size Factor", "Standard Bulk Calculations": Value Change {
        w908 = u8 2 ("Plot Interpolation")
        n617 = event-data() -> ()  [unwired: 1 in, 5 out]
        n618 = local read "All DFT Data Summary"() -> (w905:T8)
        n619 = Unbundle By Name(w905) -> ("Headers"=w903:string[], "Relaxation Data"=w904:string[][])
        n620 = for {
          tunnel: w903 -> [w938]
          tunnel: string[] ["Final_Energy_(eV)", "Net_Charge"] -> [w937] mode=indexing
          tunnel: [w936] -> w901 mode=indexing
          n621 = Search 1D Array(1D array=w938, element=w937) -> (index of element=w936:i32)  [unwired: 1 in]
        }
        n622 = Empty Array?(array="Standard Bulk Calculations") -> (empty?=w898:bool)
        n623 = Index Array(array="Standard Bulk Calculations") -> (element=w896:i32)  [unwired: 1 in]
        n624 = Index Array(array=w901) -> (element #1=w900:i32, element #2=w899:i32)  [unwired: 2 in]
        n625 = case shown="False" w898 {
          tunnel: w904 -> [_ w935]
          tunnel: w900 -> [_ w934]
          tunnel: w896 -> [w918 _]
          tunnel: [w917 w921] -> w895
          frame False {
            n626 = Index Array(array="Bulk Stds", index=w918) -> (element=w917:T32)
          }
          frame True {
            n627 = local read "Loaded DFT Paths"() -> (w929:path[])
            n628 = Index Array(array="Loaded Files") -> (element=w932:i32)  [unwired: 1 in]
            n629 = Index Array(array=w935, index (row)=w932) -> (element=w930:string[])  [unwired: 1 in]
            n630 = Index Array(array=w930, index #2=w934) -> (element #1=w922:string, element #2=w931:string)  [unwired: 1 in]
            n631 = String To Path(string=w922) -> (path=w928:path)
            n632 = Search 1D Array(1D array=w929, element=w928) -> (index of element=w926:i32)  [unwired: 1 in]
            n633 = local read "Structures"() -> (w927:T12)
            n634 = Fract/Exp String To Number(string=w931) -> (number=w924:dbl)  [unwired: 3 in, 1 out]
            n635 = Index Array(array=w927, index=w926) -> (element=w925:T5)
            n636 = call "Count Atoms in Structure.vi"("Structure"=w925) -> ("Atom Counts"=w923:T33)  [unwired: 10 in]
            n637 = Bundle("String"=w922, "", w924, "Atom Counts"=w923) -> (w921:T34)  [unwired: 1 in]
          }
        }
        n638 = local read "Selection List"() -> (w916:i32[])
        n639 = for {
          tunnel: w916 -> [w987] mode=indexing
          tunnel: [w964] -> w909 mode=indexing
          tunnel: [w974] -> w912 mode=indexing
          tunnel: [w971] -> w911 mode=indexing
          tunnel: [w970] -> w906 mode=indexing
          tunnel: w904 -> [w969]
          tunnel: w900 -> [w968]
          tunnel: w899 -> [w966]
          tunnel: w895 -> [w949]
          w939 = ""
          w980 = 1.8368 ("Start")
          n640 = Unbundle By Name(w949) -> ("Final Energy (eV)"=w947:dbl, "Atom Counts"=w948:T33)
          n641 = Index Array(array=w969, index (row)=w987) -> (element=w991:string[])  [unwired: 1 in]
          n642 = Index Array(array=w948) -> (element #1=w953:T35, element #2=w952:T35)  [unwired: 2 in]
          n643 = Unbundle By Name(w953) -> ("Total Count"=w951:i32)
          n644 = Unbundle By Name(w952) -> ("Total Count"=w950:i32)
          n645 = local read "Loaded DFT Paths"() -> (w985:path[])
          n646 = Index Array(array=w991, index #2=2 ("index"), index #3=w968, index #4=w966) -> (element #1=w990:string, element #2=w964:string, element #3=w986:string, element #4=w965:string)  [unwired: 1 in]
          n647 = String To Path(string=w990) -> (path=w981:path)
          n648 = local read "Using DB"() -> (w967:bool)
          n649 = Search 1D Array(1D array=w985, element=w981) -> (index of element=w988:i32)  [unwired: 1 in]
          n650 = case shown="True" w967 {
            tunnel: w981 -> [w994 _]
            tunnel: [w993 w995] -> w940
            tunnel: w965 -> [_ w996]
            frame False {
              n651 = call "Find Net Charge.vi"("DFT Path"=w994) -> ("Net Charge"=w993:i32)  [unwired: 8 in, 2 out]
            }
            frame True {
              n652 = Decimal String To Number(string=w996) -> (number=w995:i32)  [unwired: 2 in, 1 out]
            }
          }
          n653 = local read "Structures"() -> (w989:T12)
          n654 = Index Array(array=w989, index=w988) -> (element=w954:T5)
          n655 = call "Count Atoms in Structure.vi"("Structure"=w954) -> ("Atom Counts"=w944:T33)  [unwired: 10 in]
          n656 = Negate(x=w940) -> (-x=w941:i32)
          n657 = Index Array(array=w944) -> (element #1=w945:T35, element #2=w946:T35)  [unwired: 2 in]
          n658 = Unbundle By Name(w945) -> ("Total Count"=w943:i32)
          n659 = Unbundle By Name(w946) -> ("Total Count"=w942:i32)
          n660 = Multiply(x="Size Factor", y=w951) -> (x*y=w984:i32)
          n661 = Multiply(x="Size Factor", y=w950) -> (x*y=w982:i32)
          n662 = Multiply(x="Size Factor", y=w947) -> (x*y=w962:dbl)
          "Reference Energy (eV)" <- w962
          n663 = Subtract(x=w984, y=w943) -> (x-y=w961:i32)
          n664 = Subtract(x=w982, y=w942) -> (x-y=w960:i32)
          n665 = Fract/Exp String To Number(string=w986) -> (number=w959:dbl)  [unwired: 3 in, 1 out]
          n666 = Bundle(w959, w962, w961, w960, w941) -> (w970:cluster{dbl, dbl, i32, i32, i32})  [unwired: 1 in]
          n667 = Bundle(w939, w939, "Net Charge"=w940, w959) -> (w958:cluster{string, string, "Net Charge":i32, dbl})  [unwired: 1 in]
          n668 = Add(x=w980, y=1.5) -> (x+y=w979:dbl)
          n669 = Bundle("String"=w964, "Site Density"=1.0, w962, w961, w960) -> (w957:T36)  [unwired: 1 in]
          n670 = Build Array(w958) -> (w956:cluster{string, string, "Net Charge":i32, dbl}[])
          n671 = Bundle(w957, w956) -> (w955:T37)  [unwired: 1 in]
          n672 = call "Start and End to Array 2.vi"("Sweep Style"=enum16{"Linear Step", "Linear Pts", "Log Pts"}."Linear Pts", "Step or # Pts"=20.0, "End"=w979, "Start"=w980) -> ("Array"=w972:dbl[])  [unwired: 7 in]
          n673 = for {
            tunnel: w959 -> [_]
            tunnel: w972 -> [w1000] mode=indexing
            tunnel: [w1002] -> w975 mode=indexing
            tunnel: [w1001] -> w973 mode=indexing
            tunnel: w955 -> [w997]
            n674 = call "Calc Formation Energy from Defect Cluster.vi"("Chemical Potential"=0.0, "Fermi Level (eV)"=w1000, "Defect Data"=w997) -> ("Formation Energy (eV)"=w1002:dbl)  [unwired: 7 in, 1 out]
            n675 = call "Calc Formation Energy from Defect Cluster.vi"("Chemical Potential"=1.0, "Fermi Level (eV)"=w1000, "Defect Data"=w997) -> ("Formation Energy (eV)"=w1001:dbl)  [unwired: 7 in, 1 out]
          }
          n676 = Bundle("Array"=w972, w975) -> (w974:cluster{"Array":dbl[], dbl[]})  [unwired: 1 in]
          n677 = Bundle("Array"=w972, w973) -> (w971:cluster{"Array":dbl[], dbl[]})  [unwired: 1 in]
        }
        "Cd Rich Limit" <- w912
        "Te Rich Limit" <- w911
        "Selectd Defect Data" <- w906
        n678 = local read "Color Array Type"() -> (w913:T11)
        n679 = Array Size(array=w909) -> (size(s)=w914:i32)
        n680 = control-ref of="Te Rich Limit"() -> (w910:refnum<vi>)
        n681 = control-ref of="Cd Rich Limit"() -> (w915:refnum<vi>)
        n682 = call "Num of Colors to Color Array.vi"("# of Colors"=w914, "Color Array Type"=w913) -> ("Colors Array"=w907:u32[])  [unwired: 3 in]
        n683 = call "Format XY Plot.vi"("Plot Interpolation"=w908, "Colors Array"=w907, "Plot Names"=w909, "XY Graph Reference"=w915) -> ()  [unwired: 8 in]
        n684 = call "Format XY Plot.vi"("Plot Interpolation"=w908, "Colors Array"=w907, "Plot Names"=w909, "XY Graph Reference"=w910) -> ()  [unwired: 8 in]
      }
      event "Add to point defect DB": Value Change {
        n685 = event-data() -> ()  [unwired: 1 in, 5 out]
        n686 = local read "Standard Bulk Calculations"() -> (w1004:i32[])
        n687 = local read "All DFT Data Summary"() -> (w1018:T8)
        n688 = Index Array(array=w1004) -> (element=w1003:i32)  [unwired: 1 in]
        n689 = Empty Array?(array=w1004) -> (empty?=w1005:bool)
        n690 = Unbundle By Name(w1018) -> ("Headers"=w1008:string[], "Relaxation Data"=w1013:string[][])
        n691 = for {
          tunnel: w1008 -> [w1038]
          tunnel: [w1037] -> w1006 mode=indexing
          tunnel: string[] ["Defect Name", "Location", "DFT_ID"] -> [w1036] mode=indexing
          n692 = Search 1D Array(1D array=w1038, element=w1036) -> (index of element=w1037:i32)  [unwired: 1 in]
        }
        n693 = local read "Structures"() -> (w1016:T12)
        n694 = case shown="False" w1005 {
          tunnel: w1016 -> [_ w1031]
          tunnel: [w1020 w1030] -> w1015
          tunnel: w1013 -> [_ w1029]
          tunnel: [w1019 w1026] -> w1012
          tunnel: w1003 -> [w1022 _]
          frame False {
            n695 = local read "Bulk Stds"() -> (w1023:T1)
            n696 = Index Array(array=w1023, index=w1022) -> (element=w1021:T32)
            n697 = Unbundle By Name(w1021) -> ("Bulk Name"=w1019:string, "Structure ID"=w1020:string)
          }
          frame True {
            n698 = local read "Loaded Files"() -> (w1035:i32[])
            n699 = Index Array(array=w1035) -> (element=w1034:i32)  [unwired: 1 in]
            n700 = Index Array(array=w1029, index (row)=w1034, index (col)=0 ("disabled index (col)")) -> (element=w1024:string)
            n701 = local read "Loaded DFT Paths"() -> (w1033:path[])
            n702 = String To Path(string=w1024) -> (path=w1027:path)
            n703 = Search 1D Array(1D array=w1033, element=w1027) -> (index of element=w1032:i32)  [unwired: 1 in]
            n704 = Index Array(array=w1031, index=w1032) -> (element=w1028:T5)
            n705 = call "Create Structure ID from Structure.vi"("Structure"=w1028) -> ("Structure ID"=w1030:string)  [unwired: 10 in]
            n706 = Strip Path(path=w1027) -> (name=w1026:string)  [unwired: 1 out]
          }
        }
        n707 = local read "Selectd Defect Data"() -> (w1017:T13)
        n708 = local read "Selection List"() -> (w1014:i32[])
        n709 = for {
          tunnel: w1017 -> [w1078] mode=indexing
          tunnel: w1016 -> [w1082]
          tunnel: w1015 -> [w1077]
          tunnel: w1014 -> [w1086] mode=indexing
          tunnel: w1013 -> [w1087]
          tunnel: w1012 -> [w1070]
          tunnel: [w1062] -> w1011 mode=indexing
          tunnel: w1006 -> [w1060]
          n710 = Index Array(array=w1087, index (row)=w1086) -> (element=w1085:string[])  [unwired: 1 in]
          n711 = local read "Loaded DFT Paths"() -> (w1088:path[])
          n712 = Index Array(array=w1060) -> (element #1=w1059:i32, element #2=w1058:i32, element #3=w1057:i32)  [unwired: 3 in]
          n713 = Index Array(array=w1085, index #2=w1059, index #3=w1058, index #4=w1057) -> (element #1=w1084:string, element #2=w1064:string, element #3=w1063:string, element #4=w1056:string)  [unwired: 1 in]
          n714 = String To Path(string=w1084) -> (path=w1076:path)
          n715 = Search 1D Array(1D array=w1088, element=w1076) -> (index of element=w1081:i32)  [unwired: 1 in]
          n716 = Get Date/Time In Seconds() -> (seconds since 1Jan1904=w1069:timestamp)
          n717 = Unbundle By Name(w1078) -> ("Reference Pure Structure Energy"=w1075:dbl, "N (Cd,Ideal - Cd,Defect)"=w1074:i32, "N (Te,ideal - Te,defect)"=w1073:i32, "# Extra Electrons"=w1072:i32)  [unwired: 1 out]
          n718 = local read "Using DB"() -> (w1061:bool)
          n719 = Index Array(array=w1082, index=w1081) -> (element=w1080:T5)
          n720 = call "Timestamp to Strings.vi"("Input Time"=w1069) -> ("DB Date-Time"=w1067:string)  [unwired: 3 in, 3 out]
          n721 = Strip Path(path=w1076) -> (name=w1065:string)  [unwired: 1 out]
          n722 = case shown="True" w1061 {
            tunnel: [w1090 w1093] -> w1083
            tunnel: w1076 -> [w1089 _]
            tunnel: w1056 -> [_ w1093]
            frame False {
              n723 = Build Path(base path=w1089, name or relative path="OUTCAR") -> (appended path=w1092:path)
              n724 = call <vilib>:"MD5Checksum File.vi"("Path"=w1092) -> ("MD5 message-digest"=w1090:string)  [unwired: 9 in, 1 out]
            }
            frame True {
            }
          }
          n725 = Negate(x=w1072) -> (-x=w1071:i32)
          n726 = call "Create Structure ID from Structure.vi"("Structure"=w1080) -> ("Structure ID"=w1079:string)  [unwired: 10 in]
          n727 = Concatenate Strings(w1065, " uploaded on " ("string"), w1067) -> (w1066:string)
          n728 = Bundle("String"=w1083, "Structure ID"=w1079, "String"=w1064, "String"=w1063, w1071, "Structure ID"=w1077, "name"=w1070, "Reference Pure Structure Energy"=w1075, "N (Cd,Ideal - Cd,Defect)"=w1074, "N (Te,ideal - Te,defect)"=w1073, w1066) -> (w1062:T38)  [unwired: 1 in]
        }
        n729 = call "Verify 0D DB Entries.vi"("DB Entries"=w1011) -> ("Cancelled?"=w1009:bool, "DB Entries Out"=w1010:T39)  [unwired: 9 in]
        n730 = case shown="False" w1009 {
          tunnel: w1010 -> [w1039 _]
          frame False {
            n731 = call <vilib>:"Set Busy.vi"() -> ("error out"=w1046:errorcluster)  [unwired: 10 in, 1 out]
            n732 = call-poly <vilib>:"DB Tools Open Connection.vi"("error in (no error)"=w1046, "connection information"="Vasp DB UDL") -> ("error out"=w1042:errorcluster, "connection reference"=w1043:T22)  [unwired: 6 in]
            n733 = for {
              tunnel: w1039 -> [w1053] mode=indexing
              shift-right: [w1051] -> w1041
              shift-left: w1043 -> [w1052]
              shift-right: [w1047] -> w1040
              shift-left: w1042 -> [w1049]
              n734 = call <vilib>:"DB Tools Insert Data.vi"("data"=w1053, "table"="[0D_Point_Defects]", "connection reference"=w1052) -> ("error out"=w1048:errorcluster, "connection reference out"=w1051:T22)  [unwired: 7 in]
              n735 = Merge Errors(w1048, w1049) -> (w1047:errorcluster)
            }
            n736 = call <vilib>:"DB Tools Close Connection.vi"("error in (no error)"=w1040, "connection reference"=w1041) -> ("error out"=w1045:errorcluster)  [unwired: 5 in]
            n737 = call <vilib>:"Unset Busy.vi"("error in (no error)"=w1045) -> ()  [unwired: 10 in, 1 out]
            n738 = case shown="Error" w1045 {
              selector: w1045 -> [_ w1055]
              frame No Error {
                n739 = One Button Dialog(message="Saved!") -> ()  [unwired: 1 in, 1 out]
              }
              frame Error {
                n740 = call <vilib>:"General Error Handler.vi"("error in (no error)"=w1055) -> ()  [unwired: 10 in, 5 out]
              }
            }
          }
          frame True {
          }
        }
      }
      event "Add to README files": Value Change {
        n741 = event-data() -> ()  [unwired: 1 in, 5 out]
        n742 = call "Get Fermi Energy"() -> ("Fermi (electron) energy (eV)"=w1094:dbl)  [unwired: 17 in, 2 out]
        n743 = for {
          tunnel: string[] ["Reference Energy", "Fermi Energy (eV)", "Formation Energy (Cd Rich) (eV)", "Formation Energy (Te Rich) (eV)"] -> [w1116] mode=indexing
          tunnel: [w1115] -> w1096 mode=indexing
          tunnel: w1094 -> [w1113]
          n744 = Number To Fractional String(number=w1113, precision (6)=i16 2) -> (F-format string=w1112:string)  [unwired: 2 in]
          n745 = Concatenate Strings(w1116, " (Ef=" ("string"), w1112, ")" ("string")) -> (w1115:string)
        }
        n746 = local read "All DFT Data Summary"() -> (w1106:T8)
        n747 = Unbundle By Name(w1106) -> ("Headers"=w1105:string[], "Relaxation Data"=w1101:string[][])
        n748 = Build Array (concatenate)(w1105, w1096) -> (w1100:string[])
        n749 = local read "All Available DFT Paths"() -> (w1108:path[])
        n750 = local read "Selectd Defect Data"() -> (w1095:T13)
        n751 = Build Array (concatenate)(w1100, w1101) -> (w1104:string[][])
        n752 = local read "Selection List"() -> (w1109:i32[])
        n753 = Delete From Array(array=w1104, index (row)=0) -> (array with subset deleted=w1102:string[][])  [unwired: 2 in, 1 out]
        n754 = for {
          tunnel: w1109 -> [w1131] mode=indexing
          tunnel: w1108 -> [w1143]
          tunnel: [w1139] -> w1107
          shift-right: [w1129] -> w1099
          shift-left: w1102 -> [w1132]
          tunnel: w1100 -> [_]
          tunnel: w1101 -> [w1135]
          tunnel: w1096 -> [w1128]
          tunnel: w1095 -> [w1126] mode=indexing
          tunnel: w1094 -> [w1118]
          n755 = Index Array(array=w1143, index=w1131) -> (element=w1141:path)
          n756 = Index Array(array=w1135, index (row)=w1131) -> (element=w1134:string[])  [unwired: 1 in]
          n757 = Build Path(base path=w1141, name or relative path="README.txt") -> (appended path=w1138:path)
          n758 = Unbundle By Name(w1126) -> ("Final Total Defect Energy (eV)"=w1125:dbl, "Reference Pure Structure Energy"=w1119:dbl, "N (Cd,Ideal - Cd,Defect)"=w1124:i32, "N (Te,ideal - Te,defect)"=w1123:i32, "# Extra Electrons"=w1122:i32)
          n759 = call "Calculate Formation Energies.vi"("Fermi (electron) energy (eV)"=w1118, "# Extra Electrons"=w1122, "N (Te,ideal - Te,defect)"=w1123, "N (Cd,Ideal - Cd,Defect)"=w1124, "Reference Pure Structure Energy"=w1119, "Final Total Defect Energy (eV)"=w1125) -> ("Formation Energy (Te-Rich)"=w1120:dbl, "Formation Energy (Cd-Rich)"=w1121:dbl)  [unwired: 4 in]
          n760 = Build Array(w1119, w1118, w1121, w1120) -> (w1137:dbl[])
          n761 = Number To Fractional String(number=w1137) -> (F-format string=w1133:string[])  [unwired: 3 in]
          n762 = Build Array(w1128, w1133) -> (w1127:string[][])
          n763 = Build Array (concatenate)(w1134, w1133) -> (w1130:string[])
          n764 = Replace Array Subset(array=w1132, new element=w1130, index (row)=w1131) -> (w1129:string[][])  [unwired: 1 in]
          n765 = call-poly <vilib>:"Write To Spreadsheet File.vi"("transpose? (no:F)"=TRUE, "append to file? (new file:F)"=TRUE, "2D data"=w1127, "file path (dialog if empty)"=w1138) -> ("new file path (Not A Path if cancelled)"=w1139:path)  [unwired: 4 in]
        }
        n766 = stacked-sequence {
          tunnel: w1107 -> [_]
          frame #0 {
            n767 = One Button Dialog(message="Saved!") -> ()  [unwired: 1 in, 1 out]
          }
        }
        n768 = Bundle(w1100, w1099) -> (w1098:cluster{string[], string[][]})  [unwired: 1 in]
        n769 = local write "All DFT Data Summary"(w1098) -> ()
      }
      event "Interface Free Reference Energy", "GB Size Factor": Value Change {
        n770 = event-data() -> ()  [unwired: 1 in, 5 out]
        n771 = local read "All DFT Data Summary"() -> (w1164:T8)
        n772 = Unbundle By Name(w1164) -> ("Headers"=w1159:string[], "Relaxation Data"=w1155:string[][])
        n773 = Index Array(array="Interface Free Reference Energy") -> (element=w1149:i32)  [unwired: 1 in]
        n774 = Search 1D Array(1D array=w1159, element="Final_Energy_(eV)" ("name or relative path")) -> (index of element=w1150:i32)  [unwired: 1 in]
        n775 = Search 1D Array(1D array=w1159, element="# of interfaces" ("name or relative path")) -> (index of element=w1157:i32)  [unwired: 1 in]
        n776 = Index Array(array=w1155, index (row)=w1149, index (col)=w1150) -> (element=w1153:string)
        n777 = Fract/Exp String To Number(string=w1153) -> (number=w1152:dbl)  [unwired: 3 in, 1 out]
        n778 = local read "Loaded DFT Paths"() -> (w1162:path[])
        n779 = local read "Selection List"() -> (w1161:i32[])
        n780 = Multiply(x=w1152, y="GB Size Factor") -> (x*y=w1151:dbl)
        "GB Reference Energy (eV)" <- w1151
        n781 = local read "Structures"() -> (w1156:T12)
        n782 = for {
          tunnel: w1161 -> [w1203] mode=indexing
          tunnel: w1155 -> [w1204]
          tunnel: w1162 -> [w1201]
          tunnel: w1150 -> [w1190]
          tunnel: w1157 -> [w1189]
          tunnel: w1156 -> [w1186]
          tunnel: w1151 -> [w1180]
          tunnel: [w1168] -> w1145 mode=indexing
          w1172 = 3.81593333333333 ("y")
          w1198 = 16021.7656  # Unit Conversion
          n783 = Index Array(array=w1204, index (row)=w1203) -> (element=w1202:string[])  [unwired: 1 in]
          n784 = Index Array(array=w1202, index #1=0 ("index"), index #2=w1190, index #3=w1189) -> (element #1=w1183:string, element #2=w1188:string, element #3=w1187:string)
          n785 = String To Path(string=w1183) -> (path=w1181:path)
          n786 = Fract/Exp String To Number(string=w1188) -> (number=w1196:dbl)  [unwired: 3 in, 1 out]
          n787 = Fract/Exp String To Number(string=w1187) -> (number=w1177:dbl)  [unwired: 3 in, 1 out]
          n788 = Subtract(x=w1196, y=w1180) -> (x-y=w1200:dbl)
          n789 = Equal To 0?(x=w1177) -> (x = 0?=w1179:bool)
          n790 = Search 1D Array(1D array=w1201, element=w1181) -> (index of element=w1185:i32)  [unwired: 1 in]
          n791 = Index Array(array=w1186, index=w1185) -> (element=w1184:T5)
          n792 = Select(t=2.0, s=w1179, f=w1177) -> (s? t:f=w1176:dbl)
          n793 = Unbundle By Name(w1184) -> ("Lattice vector a"=w1194:dbl[], "Lattice vector b"=w1193:dbl[], "Lattice vector c"=w1191:dbl[])
          n794 = call <vilib>:"Cross Product.vi"("B Vector"=w1193, "A Vector"=w1194) -> ("Cross Product"=w1195:dbl[])  [unwired: 8 in, 1 out]
          n795 = call-poly <vilib>:"Vector Norm.vi"("Input Vector"=w1191) -> ("norm"=w1171:dbl)  [unwired: 9 in, 1 out]
          n796 = Divide(x=w1171, y=w1172) -> (x/y=w1173:dbl)
          n797 = call-poly <vilib>:"Vector Norm.vi"("Input Vector"=w1195) -> ("norm"=w1192:dbl)  [unwired: 9 in, 1 out]
          n798 = Divide(x=w1200, y=w1192) -> (x/y=w1199:dbl)
          n799 = Round To Nearest(number=w1173) -> (nearest integer value=w1175:dbl)
          n800 = Multiply(x=w1172, y=w1175) -> (x*y=w1174:dbl)
          n801 = Multiply(x=w1198, y=w1199) -> (x*y=w1197:dbl)
          n802 = Subtract(x=w1171, y=w1174) -> (x-y=w1170:dbl)
          n803 = Divide(x=w1197, y=w1176) -> (x/y=w1169:dbl)
          n804 = Bundle(w1170, w1169) -> (w1168:cluster{dbl, dbl})  [unwired: 1 in]
        }
        n805 = Sort 1D Array(array=w1145) -> (sorted array=w1148:cluster{dbl, dbl}[])
        n806 = for {
          tunnel: w1148 -> [w1167] mode=indexing
          tunnel: [w1166] -> w1147 mode=indexing
          tunnel: [w1165] -> w1146 mode=indexing
          n807 = Unbundle(w1167) -> (w1166:dbl, w1165:dbl)
        }
        n808 = Bundle(w1147, w1146) -> (→"GB Bivariate Plot":cluster{dbl[], dbl[]})  [unwired: 1 in]
      }
      event "Add to GB DB": Value Change {
        n809 = event-data() -> ()  [unwired: 1 in, 5 out]
        n810 = local read "Interface Free Reference Energy"() -> (w1208:i32[])
        n811 = local read "All DFT Data Summary"() -> (w1226:T8)
        n812 = Unbundle By Name(w1226) -> ("Headers"=w1229:string[], "Relaxation Data"=w1207:string[][])
        n813 = Index Array(array=w1208) -> (element=w1212:i32)  [unwired: 1 in]
        n814 = local read "Loaded DFT Paths"() -> (w1211:path[])
        n815 = for {
          tunnel: w1229 -> [w1233]
          tunnel: [w1232] -> w1214 mode=indexing
          tunnel: string[] ["Folder", "# of interfaces", "Final_Energy_(eV)", "GB_dof_ID", "DFT_ID"] -> [w1231] mode=indexing
          n816 = Search 1D Array(1D array=w1233, element=w1231) -> (index of element=w1232:i32)  [unwired: 1 in]
        }
        n817 = Index Array(array=w1207, index (row)=w1212, index (col)=0 ("disabled index (col)")) -> (element=w1209:string)
        n818 = String To Path(string=w1209) -> (path=w1205:path)
        n819 = local read "Structures"() -> (w1225:T12)
        n820 = Search 1D Array(1D array=w1211, element=w1205) -> (index of element=w1206:i32)  [unwired: 1 in]
        n821 = local read "GB Reference Energy (eV)"() -> (w1213:dbl)
        n822 = local read "Loaded DFT Paths"() -> (w1228:path[])
        n823 = local read "Vasp DB UDL"() -> (w1227:path)
        n824 = local read "Selection List"() -> (w1223:i32[])
        n825 = Index Array(array=w1225, index=w1206) -> (element=w1222:T5)
        n826 = call <vilib>:"Set Busy.vi"() -> ("error out"=w1216:errorcluster)  [unwired: 10 in, 1 out]
        n827 = call "Create Structure ID from Structure.vi"("Structure"=w1222) -> ("Structure ID"=w1224:string)  [unwired: 10 in]
        n828 = Strip Path(path=w1205) -> (name=w1217:string)  [unwired: 1 out]
        n829 = call-poly <vilib>:"DB Tools Open Connection.vi"("error in (no error)"=w1216, "connection information"=w1227) -> ("error out"=w1219:errorcluster, "connection reference"=w1221:T22)  [unwired: 6 in]
        n830 = for {
          tunnel: w1225 -> [w1291]
          tunnel: w1224 -> [w1274]
          tunnel: w1223 -> [w1295] mode=indexing
          tunnel: w1207 -> [w1296]
          shift-right: [w1286] -> w1220
          shift-left: w1221 -> [w1287]
          shift-right: [w1282] -> w1218
          shift-left: w1219 -> [w1283]
          tunnel: w1217 -> [w1273]
          tunnel: w1228 -> [w1275]
          tunnel: w1213 -> [w1267]
          tunnel: w1214 -> [w1258]
          w1244 = 3.81593333333333 ("y")
          w1269 = 16021.7656  # Unit Conversion
          n831 = Index Array(array=w1296, index (row)=w1295) -> (element=w1294:string[])  [unwired: 1 in]
          n832 = Index Array(array=w1258) -> (element #1=w1257:i32, element #2=w1256:i32, element #3=w1255:i32, element #4=w1254:i32, element #5=w1237:i32)  [unwired: 5 in]
          n833 = Index Array(array=w1294, index #2=w1257, index #3=w1256, index #4=w1255, index #5=w1254, index #6=w1237) -> (element #1=w1293:string, element #2=w1276:string, element #3=w1272:string, element #4=w1266:string, element #5=w1240:string, element #6=w1236:string)  [unwired: 1 in]
          n834 = String To Path(string=w1293) -> (path=w1288:path)
          n835 = case shown="\"\"" w1236 {
            selector: w1236 -> [w1297 _]
            tunnel: [w1297 w1299] -> w1292
            tunnel: w1288 -> [_ w1298]
            frame Default {
            }
            frame "" {
              n836 = Build Path(base path=w1298, name or relative path="OUTCAR") -> (appended path=w1301:path)
              n837 = call <vilib>:"MD5Checksum File.vi"("Path"=w1301) -> ("MD5 message-digest"=w1299:string)  [unwired: 9 in, 1 out]
            }
          }
          n838 = Fract/Exp String To Number(string=w1272) -> (number=w1249:dbl)  [unwired: 3 in, 1 out]
          n839 = Fract/Exp String To Number(string=w1266) -> (number=w1265:dbl)  [unwired: 3 in, 1 out]
          n840 = Search 1D Array(1D array=w1275, element=w1288) -> (index of element=w1290:i32)  [unwired: 1 in]
          n841 = Subtract(x=w1265, y=w1267) -> (x-y=w1271:dbl)
          n842 = Equal To 0?(x=w1249) -> (x = 0?=w1251:bool)
          n843 = Index Array(array=w1291, index=w1290) -> (element=w1264:T5)
          n844 = Select(t=2.0, s=w1251, f=w1249) -> (s? t:f=w1248:dbl)
          n845 = Empty String/Path?(string/path=w1240) -> (empty?=w1241:bool)
          n846 = Unbundle By Name(w1264) -> ("Lattice vector a"=w1262:dbl[], "Lattice vector b"=w1261:dbl[], "Lattice vector c"=w1253:dbl[])
          n847 = Select(t="1", s=w1241, f=w1240) -> (s? t:f=w1238:string)
          n848 = call "Create Structure ID from Structure.vi"("Structure"=w1264) -> ("Structure ID"=w1289:string)  [unwired: 10 in]
          n849 = call <vilib>:"Cross Product.vi"("B Vector"=w1261, "A Vector"=w1262) -> ("Cross Product"=w1263:dbl[])  [unwired: 8 in, 1 out]
          n850 = call-poly <vilib>:"Vector Norm.vi"("Input Vector"=w1253) -> ("norm"=w1243:dbl)  [unwired: 9 in, 1 out]
          n851 = Divide(x=w1243, y=w1244) -> (x/y=w1245:dbl)
          n852 = call-poly <vilib>:"Vector Norm.vi"("Input Vector"=w1263) -> ("norm"=w1260:dbl)  [unwired: 9 in, 1 out]
          n853 = Divide(x=w1271, y=w1260) -> (x/y=w1270:dbl)
          n854 = Round To Nearest(number=w1245) -> (nearest integer value=w1247:dbl)
          n855 = Get Date/Time In Seconds() -> (seconds since 1Jan1904=w1281:timestamp)
          n856 = Multiply(x=w1269, y=w1270) -> (x*y=w1268:dbl)
          n857 = Multiply(x=w1244, y=w1247) -> (x*y=w1246:dbl)
          n858 = call "Timestamp to Strings.vi"("Input Time"=w1281) -> ("DB Date-Time"=w1279:string)  [unwired: 3 in, 3 out]
          n859 = Strip Path(path=w1288) -> (name=w1277:string)  [unwired: 1 out]
          n860 = Divide(x=w1268, y=w1248) -> (x/y=w1259:dbl)
          n861 = Subtract(x=w1243, y=w1246) -> (x-y=w1242:dbl)
          n862 = Concatenate Strings(w1277, " uploaded on " ("string"), w1279) -> (w1278:string)
          n863 = Bundle("MD5 message-digest"=w1292, "Structure ID"=w1289, "String"=w1276, "Structure ID"=w1274, "name"=w1273, "GB Reference Energy (eV)"=w1267, "t"=w1248, w1259, w1242, "String"=w1238, w1278) -> (w1252:T40)  [unwired: 1 in]
          n864 = call <vilib>:"DB Tools Insert Data.vi"("data"=w1252, "table"="[2D_Grain_Boundaries]", "connection reference"=w1287) -> ("error out"=w1284:errorcluster, "connection reference out"=w1286:T22)  [unwired: 7 in]
          n865 = Merge Errors(w1284, w1283) -> (w1282:errorcluster)
        }
        n866 = call <vilib>:"DB Tools Close Connection.vi"("error in (no error)"=w1218, "connection reference"=w1220) -> ("error out"=w1215:errorcluster)  [unwired: 5 in]
        n867 = call <vilib>:"Unset Busy.vi"("error in (no error)"=w1215) -> ()  [unwired: 10 in, 1 out]
        n868 = case shown="Error" w1215 {
          selector: w1215 -> [_ w1235]
          frame No Error {
            n869 = One Button Dialog(message="Saved!") -> ()  [unwired: 1 in, 1 out]
          }
          frame Error {
            n870 = call <vilib>:"General Error Handler.vi"("error in (no error)"=w1235) -> ()  [unwired: 10 in, 5 out]
          }
        }
      }
    }
  }
  n871 = call <vilib>:"Create Object.vi"("Name"="Base") -> ("Scene:New Object"=w1:refnum<vi>)  [unwired: 1 in, 9 out]
  n872 = local write "Base Object"(w1) -> ()
